vi "IMAQController.panel2.vi"(0 "object ref":refnum<vi>, 5 "error in (no error)":errorcluster) -> ()   [LabVIEW 2014]
doc: "This is the front panel VI for the PTScanner class.\n\ndescriptionHelpStart\nThe PTScanner class has been designed to be used interactively by a normal user. The main aim of this class is to provide a possibility of multi-dimensional scan for any integer or floating-point single value among the CS system.\n\nAt first, user has to add values to be scanned and to organize them in the corresponding order. Each value is represented by several parameters:\n- object\n- \"set\" method (can have many parameters)\n- method parameters (with one of them to be scanned)\n- central point\n- \"minus\" and \"plus\" values (start point is a difference between \"central\" and \"minus\" values, stop point is a sum of \"central\" and \"plus\" respectively)\n- step size\n- call mode which means how will be realized the movement from one step to the next one. The check of nominal (from current step) and actual values conformity can be done in a simple mode (here you should know the corresponding service) or in a synchronous mode (assuming that the method has a feedback of excatly the same parameters as input parameters)\n- as an option one can input service address for the synchronization directly. Do it only if you know exactly what is it!!!\n\nAfter the list of values is formed you have to form the scan sequence. You can check the scan sequence by \"View -> Scan Table\" from the window menu (have to wait some time before the representation table will be formed). Now you can run your scan in two modes: single (sequence will be runned only once) and loop (sequence will be runned continuously).\n\nDelay is a delay time (in ms) between two steps.\ndescriptionHelpStop\n\nLicense Agreement for the PTScanner class:\n\nCopyright (C)\nMikhail Goncharov\nMax-Planck-Institut fuer Kernphysik\nSaupfercheckweg 1\n69117 Heidelberg\nGermany\n\nContact: mikhail.goncharov@mpi-hd.mpg.de\n\nThis program is free software; you can redistribute it and/or modify it under the terms of the GNU General Public License as published by the Free Software Foundation; either version 2 of the license, or (at your option) any later version.\n\nThis program is distributed in the hope that it will be useful, but WITHOUT ANY WARRANTY; without even the implied warranty of MERCHANTABILITY or FITNESS FOR A PARTICULAR PURPOSE. See the GNU General License for more details (http://www.gnu.org).\n\nLast update: 2-DEC-2010\n\n\nmenuHelpStart\nFile\n==\n- \"Load\" loads a list of values to be scanned. After that you have to form a scan.\n\n- \"Save/Save As\" saves the actual list of values.\n\n- \"Hide\" just hides this GUI (but it remains alive in the background).\n\n- \"Close\" closes this window and removes this process from the system.\n\nOperate\n=====\n- \"Start\" starts scan sequence. Awailable only after the sequence is formed.\n\n- \"Pause\" pauses current run. Awailable only during the running of the sequence.\n\n- \"Stop\" stops scan sequence.\n\n- \"Reset\" resets the scanner (sets the first step as a current and nulls all counters).\n\n- \"Reset Values\" sets all variables to their central values.\n\nView\n=====\n- \"Scan Table\" forms and shows the representation of the current formed scan sequence. If there are a lot of steps and values it could take some time so be patient =)\nmenuHelpStop"
uses:
  CSlibraries-extern/DimLVEvent/DimIndicators/DimIndicators.lvlib
  CSCore/CSSystem/CSSystemLib/CSSystemLib.lvlib
  CSlibraries-extern/DimLVEvent/LVDimInterface/LVDimInterface.lvlib
  CSlibraries-extern/DimLVEvent/LVDimInterface/LVDimInterface.dim service type.ctl
  CSlibraries-extern/DimLVEvent/LVDimInterface/LVDimInterface.dic_info_service_notifier.vi
  CSCore/CSObj/CSObj.lvlib
  IMAQController.lvlib
  CSCore/BaseProcess/BaseProcess.lvlib
  CSCore/CSSystem/CoreLib/CoreLib.lvlib
  CSCore/CSSystem/CoreLib/CoreLib.short 2 byte array.vi
  CSlibraries-extern/HGF/HGF_VisionTools/HGF_VisionTools.lvlib
  CSlibraries-extern/DimLVEvent/LVDimInterface/LVDimInterface.dic_info_service_queue.vi
  CSlibraries-extern/DimLVEvent/DimIndicators/DimIndicators.numericType.ctl
  CSlibraries-extern/DimLVEvent/DimIndicators/DimIndicators.anyType.ctl
  CSlibraries-extern/DimLVEvent/DimIndicators/DimIndicators.numericArrayType.ctl
panel:
  out "Image hight":i32
  out "Image length":i32
  out "receivedCounter":i32
  out "receivedCounter 2":i32
  out "aktueller\nService":i32
  out "callBackID":i32
  out "no link":bool
  out "DIM service length / byte":i32
  out "act Time Stamp":i16[](array[numeric])
  out "2nd loop":i32
  out "accepted update 2nd loop":i32
  out "error out 3":errorcluster
  in  "error out 2":errorcluster
  out "TimeStamp Data":i16[](array[numeric])
  out "Abbruch durch Asynch":bool
  out "Abbruch?":bool
  out "accepted updates?":i32
  out "updates?":i32
  out "TimeStamp Analyzer":i16[](array[numeric])
  out "Data Ana Synch?":bool
  out "floor(x/y)":i32
  in  "Limits (L:0,H:255)":cluster{u8, u8}(slide)={0, 255} scale=0.0..255.0
  in  "Grab":bool
  in  "Snap":bool
  in  "Compression mode?":bool
  out "Busy 3":bool
  out "Busy 2":bool
  in  "IMAQDevice Mode":u16(ring) caption="IMAQDevice:" items=["cam1", "cam2"]
  in  "IMAQAnalyzer:":string
  in  "NumberOfImagesLink":T1
  out "CSNodes":string[](array[string])
  out "CSSystems":string[](array[string])
  in  "TimeStampAnalyzerLink":T2
  in  "TimeStampDeviceLink":T2
  in  "IntensityLink":T1
  in  "verticalProjectionLink":T2
  in  "horizontalProjectionLink":T2
  in  "WidthLink":T1
  in  "HeightLink":T1
  in  "ActualImageLink(Compression Mode)":T3
  in  "CompressionModeLink":T1
  in  "Abort Button":bool
  in  "Stop Button":bool
  in  "Start Button":bool
  in  "Step 2":dbl caption="Step"
  in  "Dec 2":dbl caption="-"
  in  "Inc 2":dbl caption="+"
  in  "Center 2":dbl caption="Center:"
  in  "Parameter 2":u16(ring) caption="Parameter:" items=["Voltage", "Current"]
  in  "Device 2":u16(ring) caption="Device:" items=["PowerSupply 1", "Power Supply 2"]
  in  "Step 1":dbl caption="Step"
  in  "Dec 1":dbl caption="-"
  in  "Inc 1":dbl caption="+"
  in  "Center 1":dbl caption="Center:"
  in  "Parameter 1":u16(ring) caption="Parameter:" items=["Voltage", "Current"]
  in  "Device 1":u16(ring) caption="Device:" items=["PowerSupply 1", "Power Supply 2"]
  in  "Scan?":bool
  in  "2 D?":bool
  in  "GetControl":bool
  out "Controller Listbox":i32(listbox)
  out "Scan_Image":T4(plugin-control)
  out "Actual_Image":T4(plugin-control)
  in  "stop":bool
  out "loop counter":i32
  out "Paused":bool
  in  "settings path":path caption="Settings file"
  out "Error":bool
  out "ErrorString":string
  out "error out":errorcluster
  # "IMAQ Configuration"
  # "Analysis Configuration"
  # "Controller Configuration"
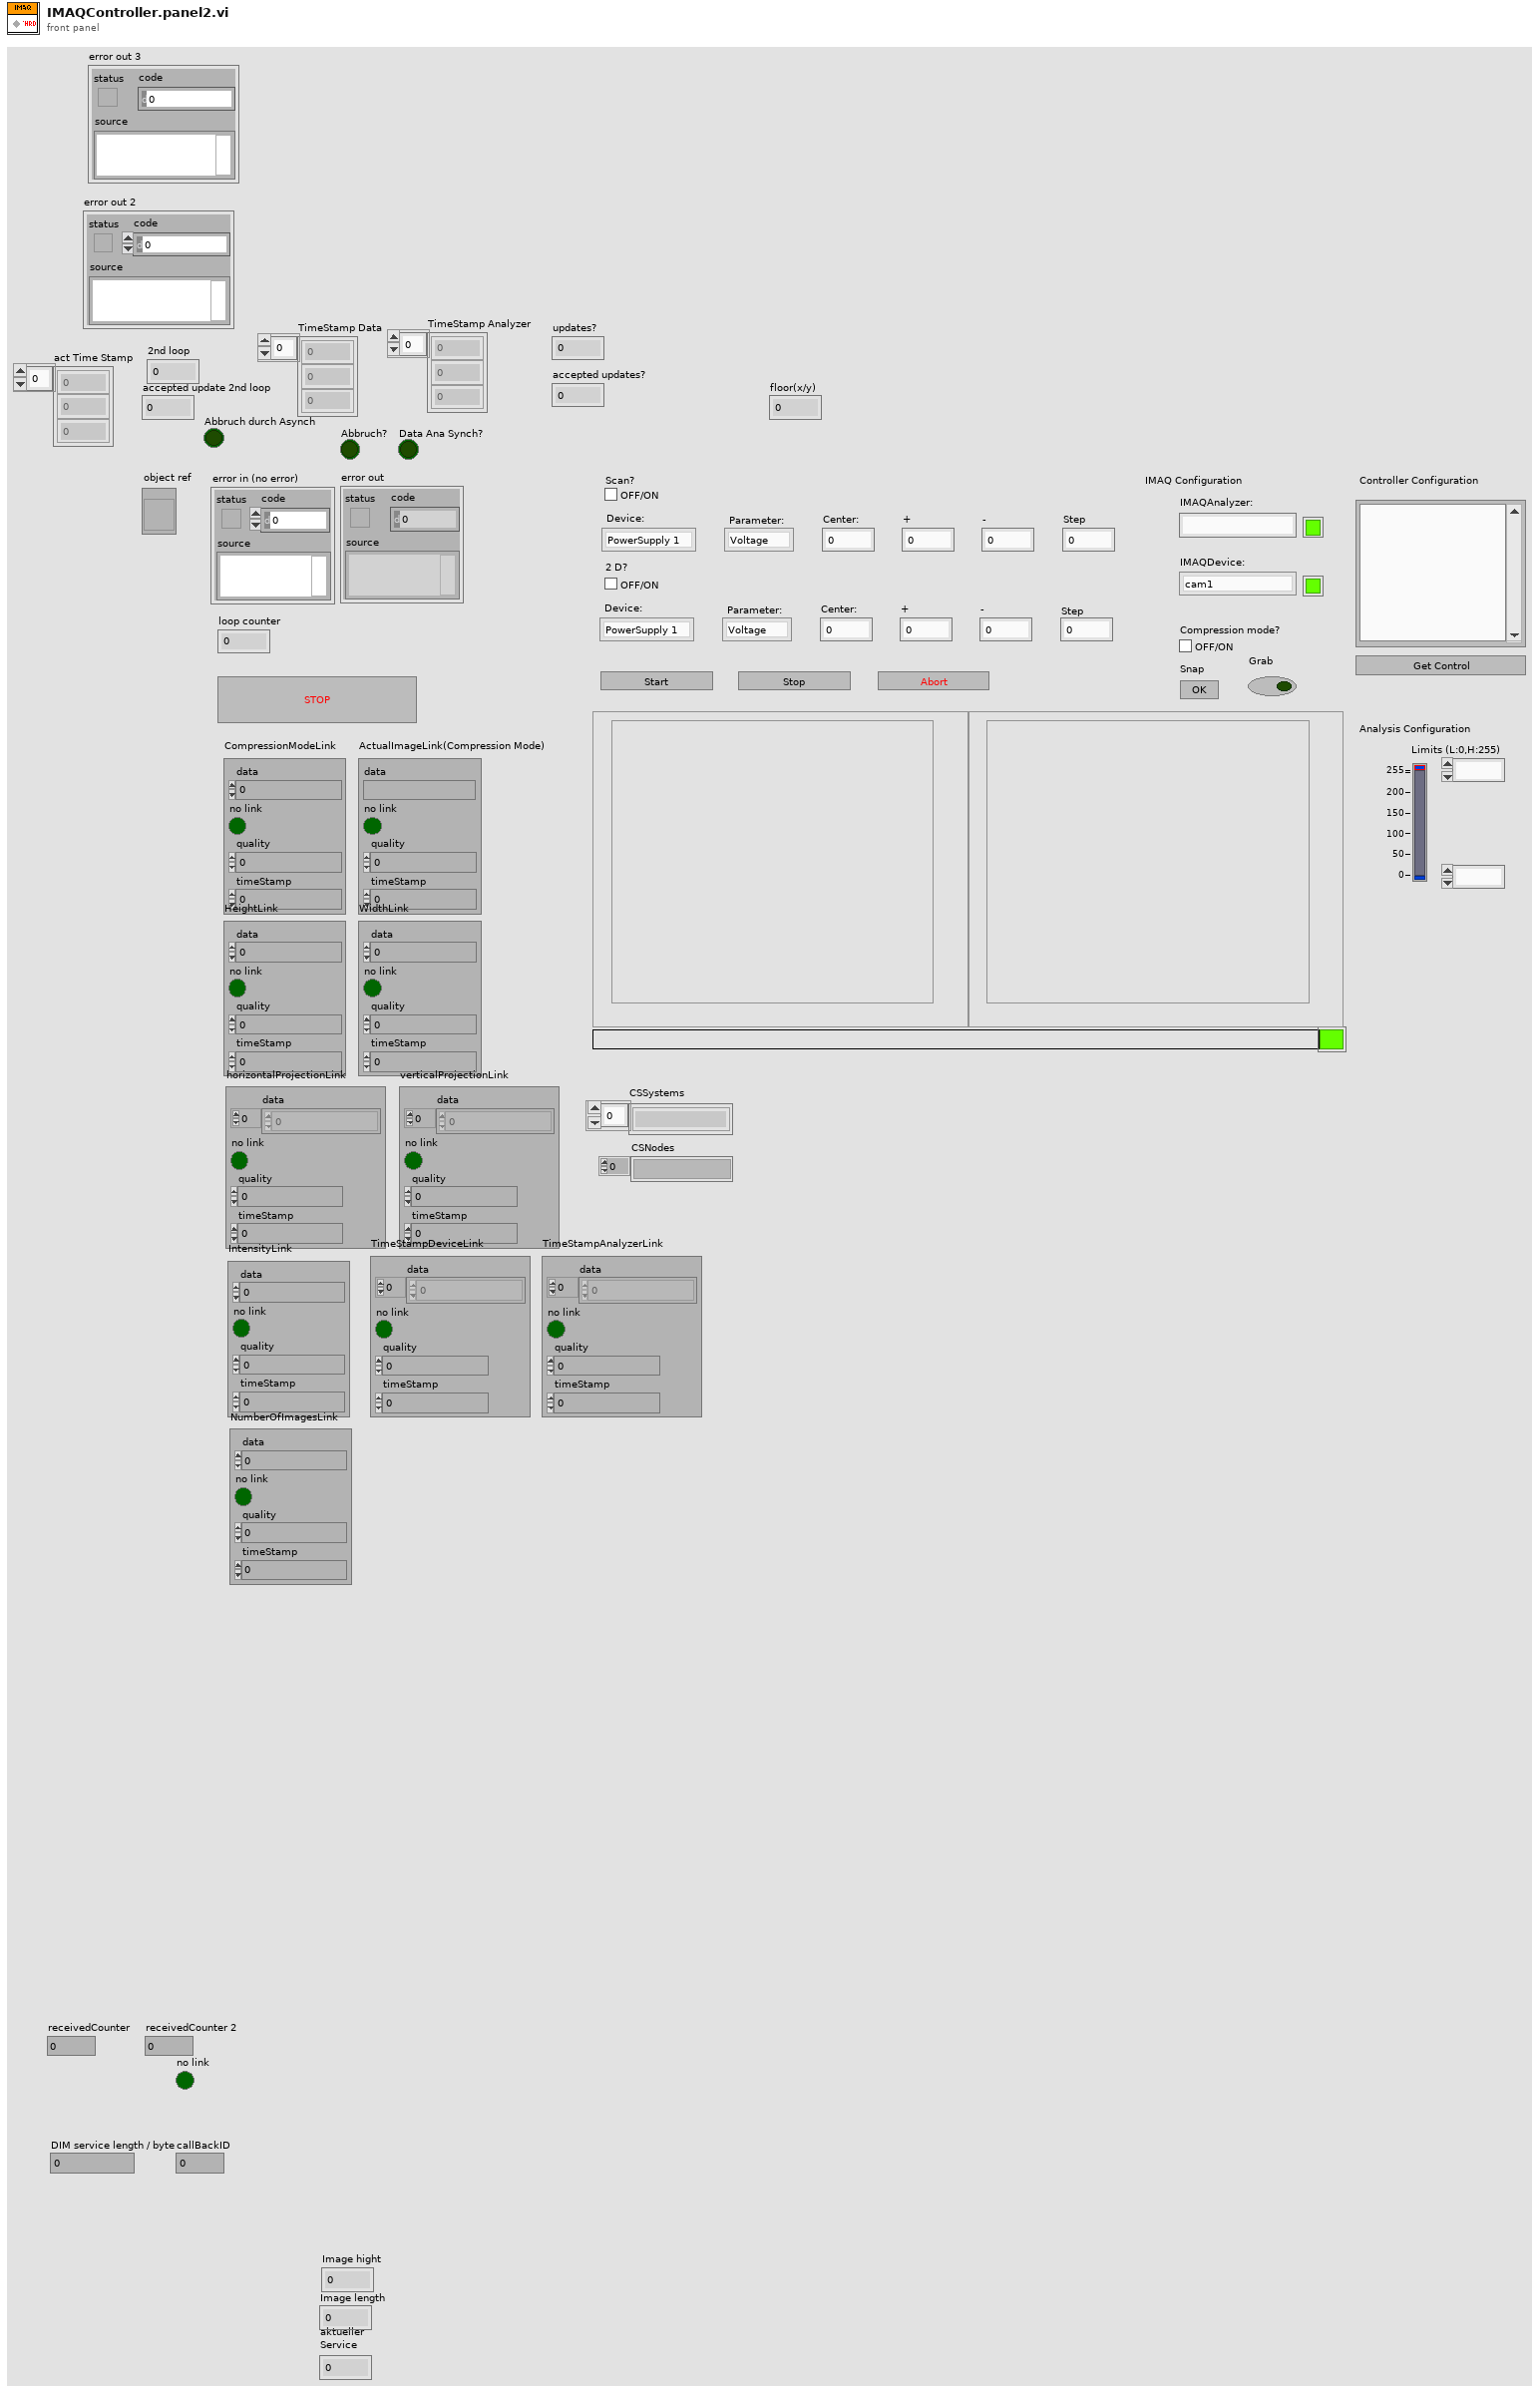
[diagram p1: front panel]
types:
  T1 = typedef "DimIndicators.lvlib/DimIndicators.numericType.ctl" = cluster{"data":dbl, "no link":bool, "quality":i32, "timeStamp":dbl}
  T2 = typedef "DimIndicators.lvlib/DimIndicators.numericArrayType.ctl" = cluster{"data":dbl[], "no link":bool, "quality":i32, "timeStamp":dbl}
  T3 = typedef "DimIndicators.lvlib/DimIndicators.anyType.ctl" = cluster{"data":string, "no link":bool, "quality":i32, "timeStamp":dbl}
  T4 = typedef "IMAQ Image.ctl" = refnum<image>
  T5 = typedef "Image Type" = u32
  T6 = typedef "IMAQController.lvlib/IMAQController.i attribute.ctl" = cluster{"ImageTakenID":i32, "actSequencer":string, "actScanner":string, "CameraTriggerID":i32, "activatedCameras":cluster{"Name":string, "Camera Type":string, "Acquisition Mode":u32, "JPEG Mode?":bool, "Acquisition Delay":dbl, "Save Images?":bool, "Center Coordinates":T7, "PixelPermm":cluster{"Horizontal":dbl, "Vertical":dbl}, "Rotation":dbl, "Mirror Mode":u32, "PixelCoordinates":cluster{"1":cluster{"Horizontal":i32, "Vertical":i32}, "2":cluster{"Horizontal":i32, "Vertical":i32}, "3":cluster{"Horizontal":i32, "Vertical":i32}, "4":cluster{"Horizontal":i32, "Vertical":i32}}, "RWCoordinates":cluster{"1":cluster{"Horizontal":dbl, "Vertical":dbl}, "2":cluster{"Horizontal":dbl, "Vertical":dbl}, "3":cluster{"Horizontal":dbl, "Vertical":dbl}, "4":cluster{"Horizontal":dbl, "Vertical":dbl}}, "HorizScaling":dbl, "VertScaling":dbl}[], "Ini C-Array":string[], "actCamera":string, "activeCamera":cluster{"Name":string, "Camera Type":string, "Aqcuisation Mode":enum32{"Internal Trigger", "Scan", "free Running", "External Trigger"}, "JPEG Mode?":bool, "Acquisition Delay":dbl, "Save Images?":bool, "Center Coordinates":T7, "PixelPermm":cluster{"Horizontal":dbl, "Vertical":dbl}, "Rotation":dbl, "Mirror Mode":u32, "PixelCoordinates":cluster{"1":cluster{"Horizontal":i32, "Vertical":i32}, "2":cluster{"Horizontal":i32, "Vertical":i32}, "3":cluster{"Horizontal":i32, "Vertical":i32}, "4":cluster{"Horizontal":i32, "Vertical":i32}}, "RWCoordinates":cluster{"1":cluster{"Horizontal":dbl, "Vertical":dbl}, "2":cluster{"Horizontal":dbl, "Vertical":dbl}, "3":cluster{"Horizontal":dbl, "Vertical":dbl}, "4":cluster{"Horizontal":dbl, "Vertical":dbl}}, "HorizScaling":dbl, "VertScaling":dbl}, "BilderMittelungen":u8, "OldPicture":dbl[][]}
  T7 = typedef "LVPoint32TypeDef.ctl" = cluster{"Horizontal":i32, "Vertical":i32}
  T8 = enum8{"Enabled", "Disabled", "Disabled and Grayed Out"}
  T9 = typedef "LVDimInterface.lvlib/LVDimInterface.dim service type.ctl" = u16
  T10 = typedef "CoreDefs.rawDataType.ctl" = i8[]
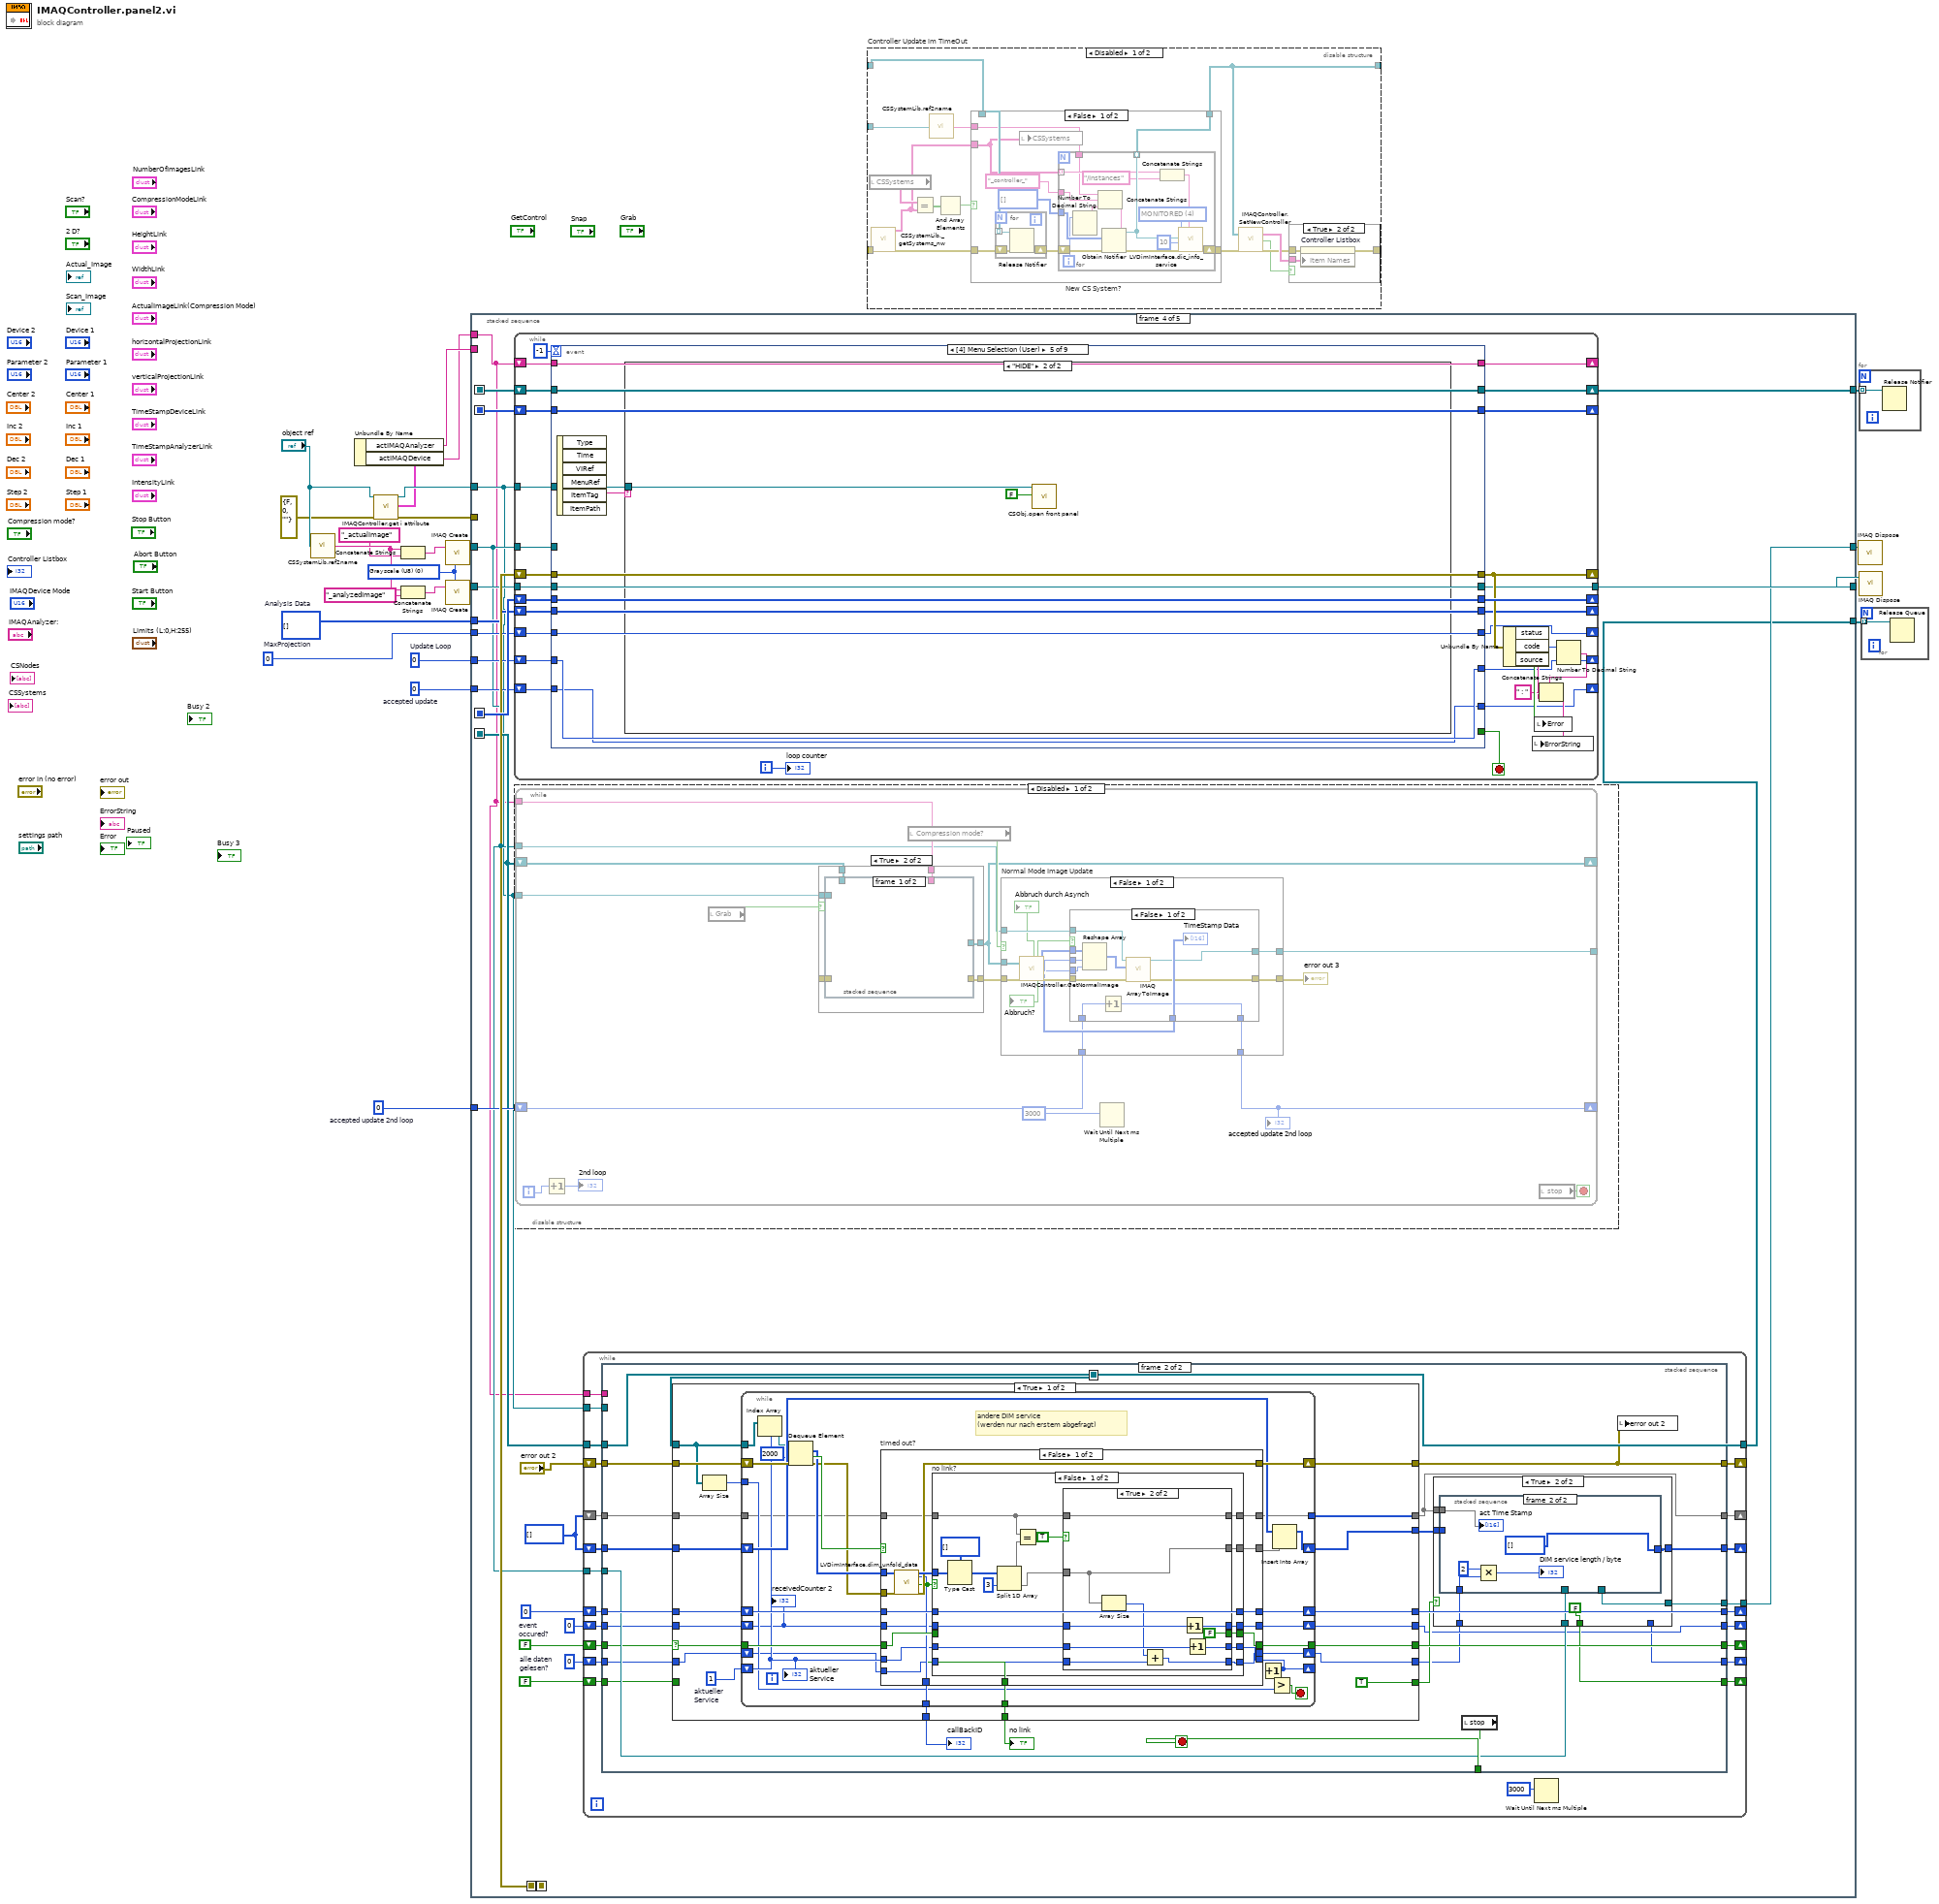
[diagram p0: block diagram]
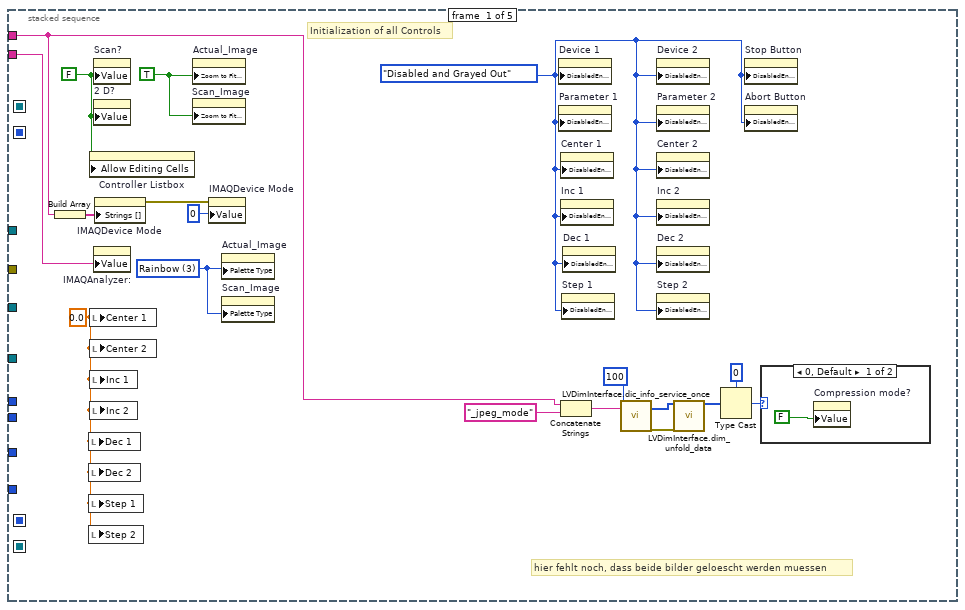
[diagram p5: hidden frame]
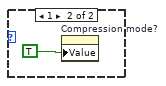
[diagram p6: hidden frame]
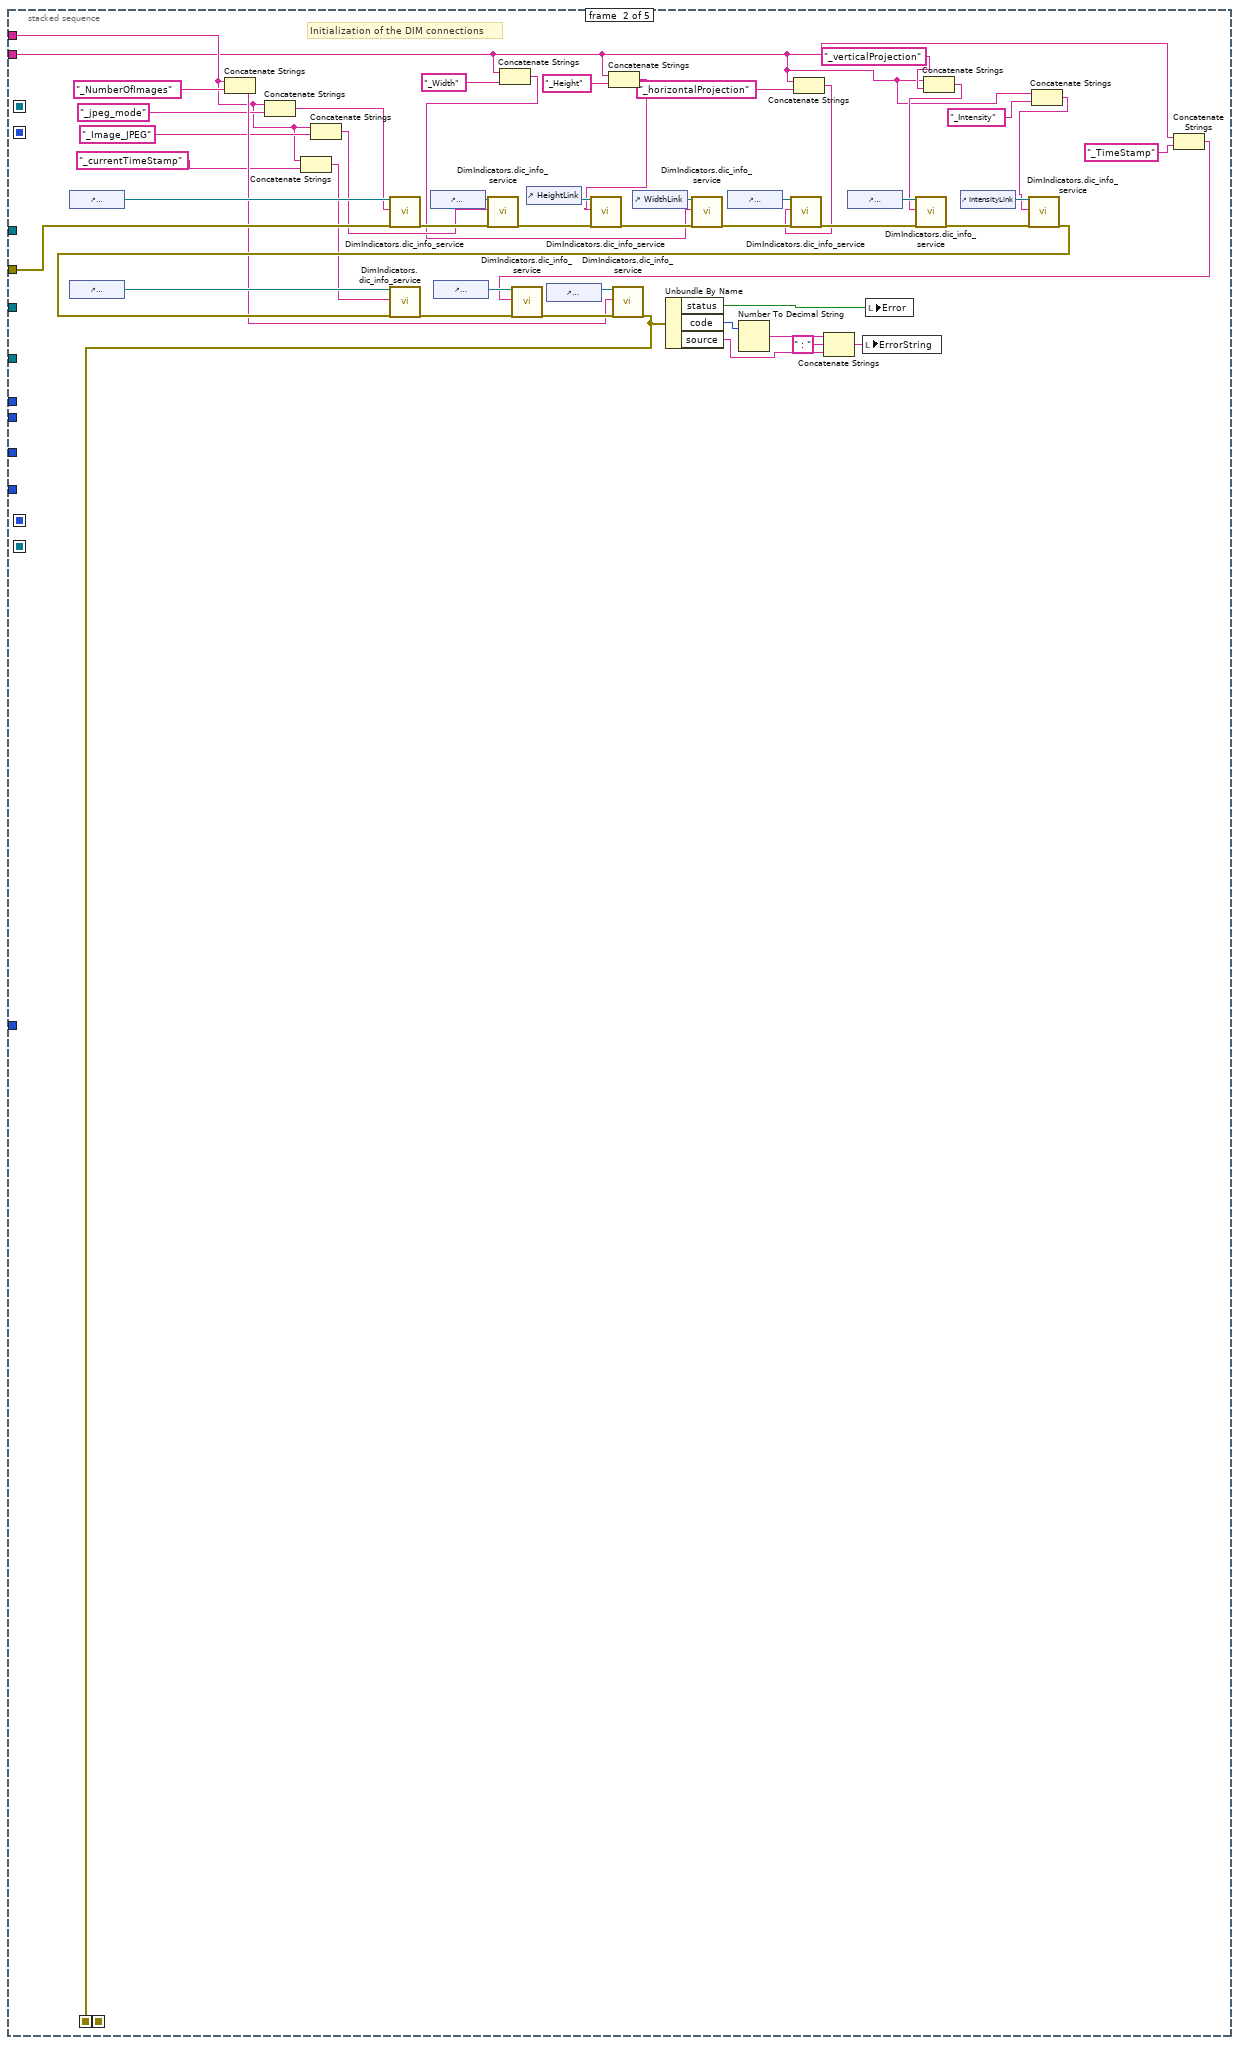
[diagram p7: hidden frame]
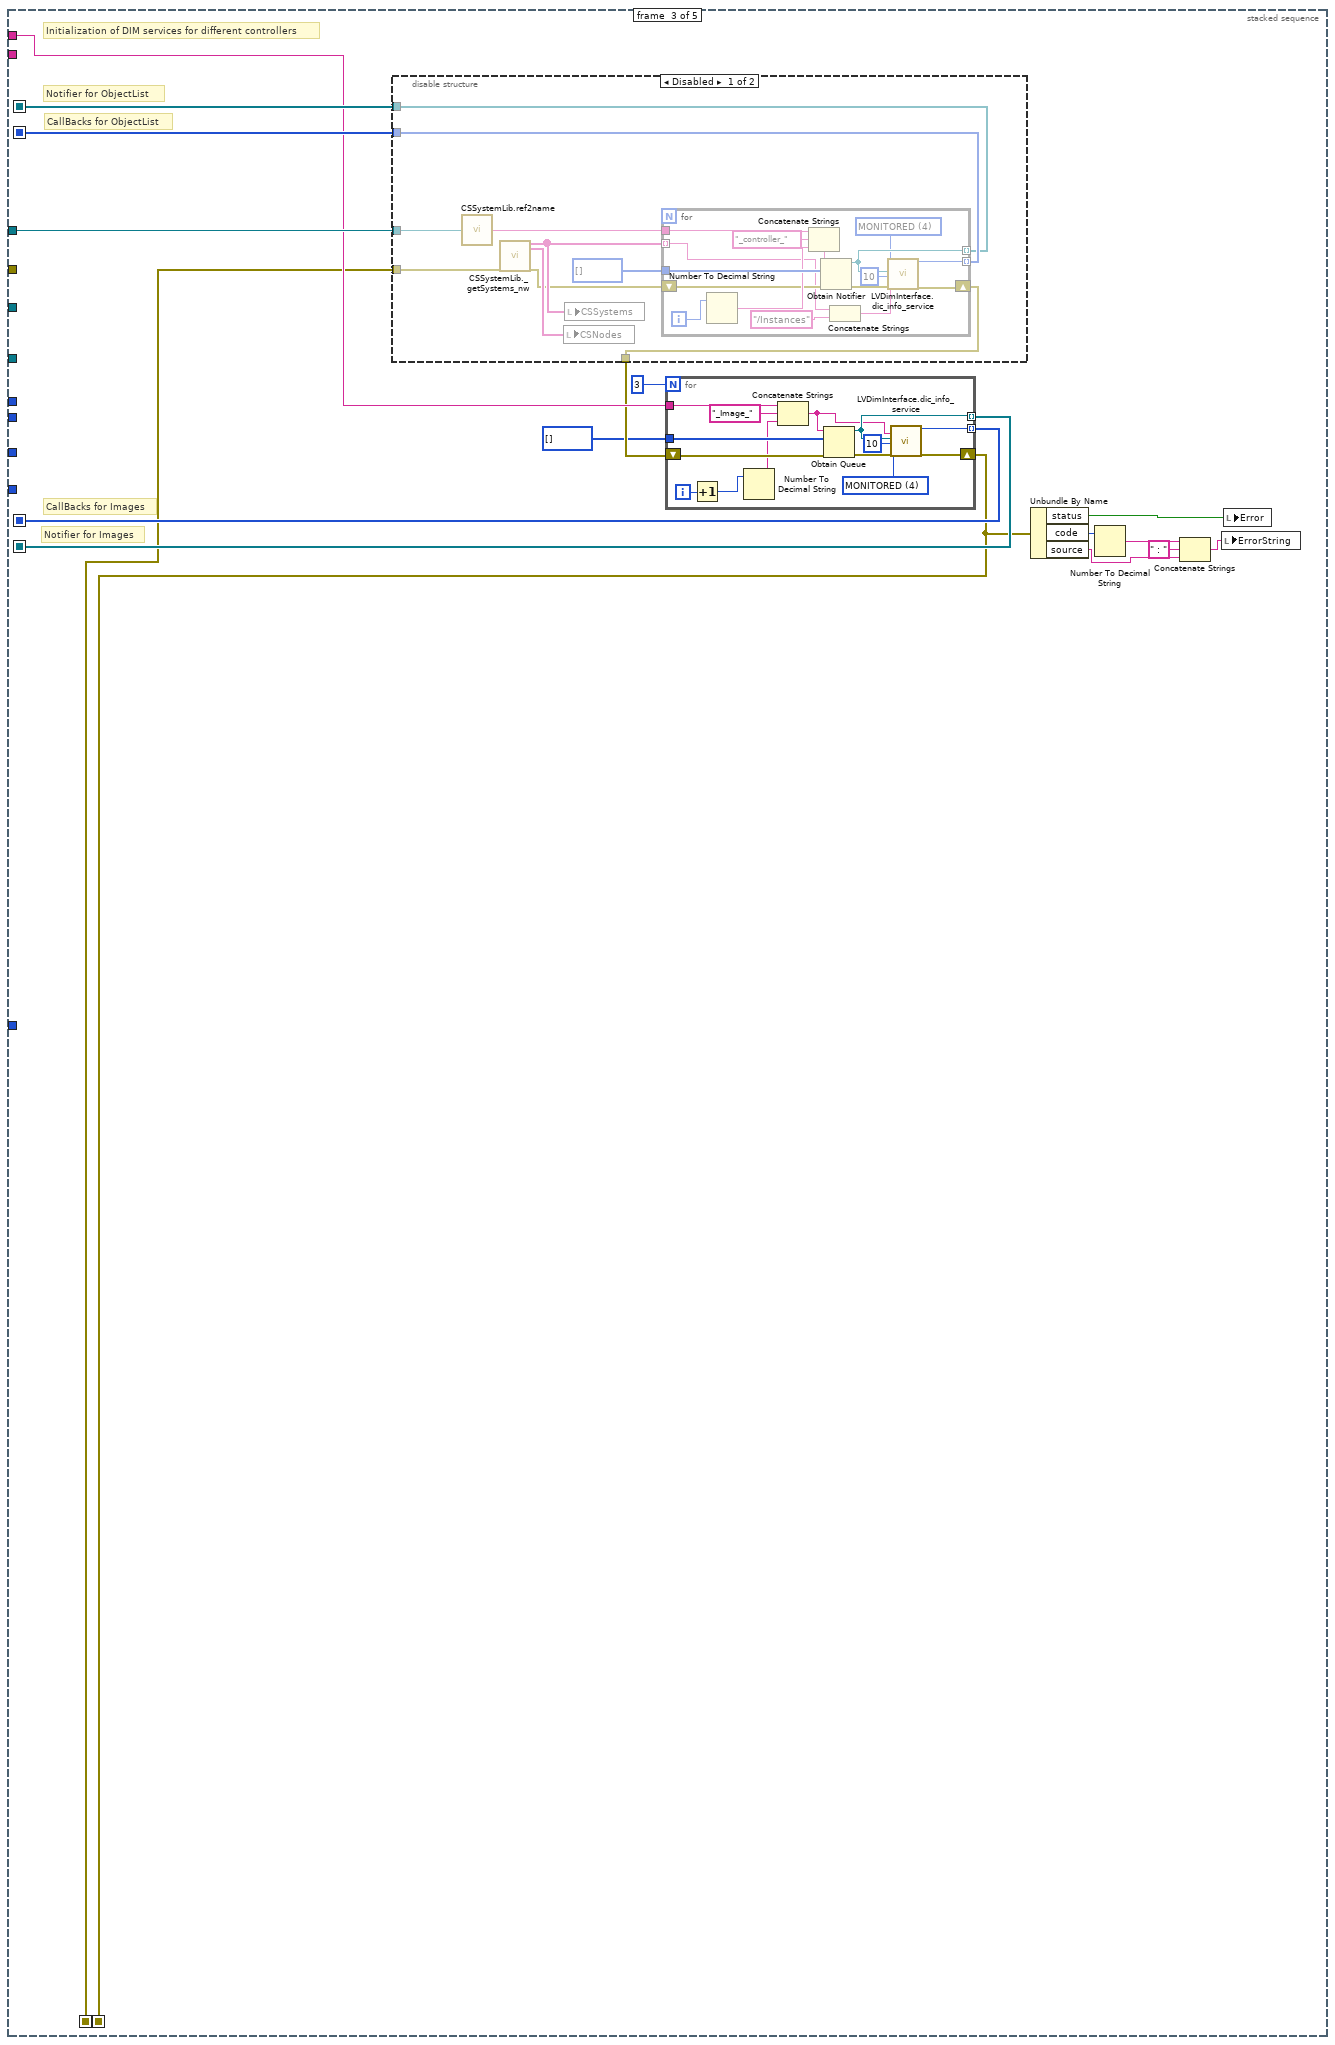
[diagram p8: hidden frame]
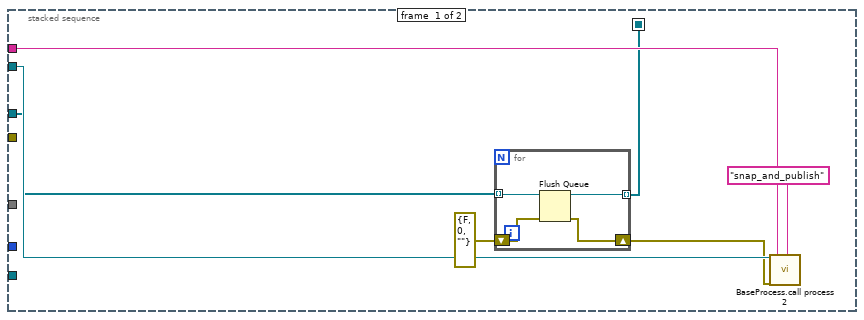
[diagram p10: hidden frame]
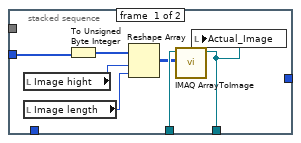
[diagram p12: hidden frame]
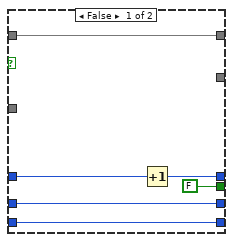
[diagram p13: hidden frame]
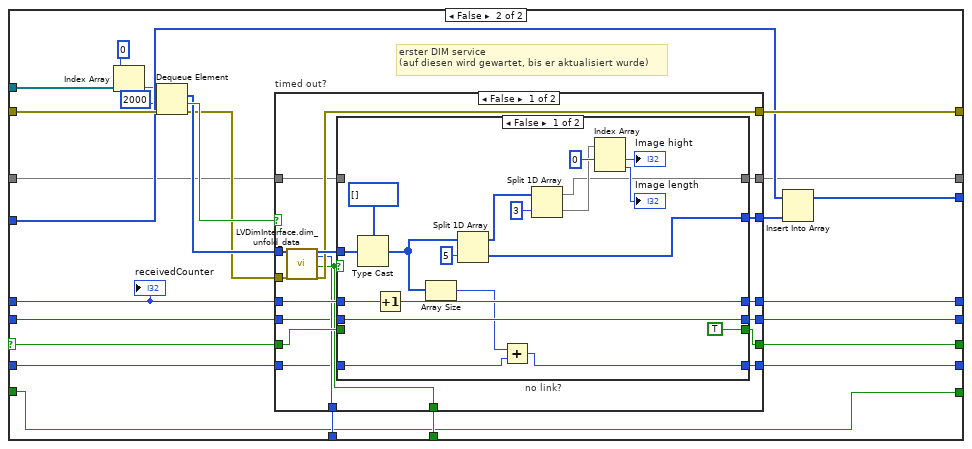
[diagram p16: hidden frame]
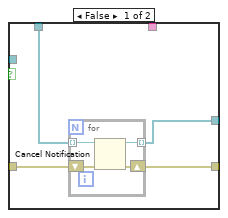
[diagram p19: hidden frame]
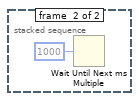
[diagram p20: hidden frame]
diagram:
  w1 = 0  # accepted update 2nd loop
  w5 = 0  # accepted update
  w4 = 0  # Update Loop
  w6 = 0  # MaxProjection
  w7 = u8[][] []  # Analysis Data
  w24 = T5 0 items=["Grayscale (U8)", "Grayscale (I16)", "Grayscale (SGL)", "Complex (CSG)", "RGB (U32)", "HSL (U32)", "RGB (U64)", "Grayscale (U16)"] ("Image Type")
  n1 = call "CSSystemLib.ref2name.vi"("obj refnum"="object ref") -> ("name"=w21:string)
  n2 = call "IMAQController.get i attribute.vi"("i ref in"="object ref", "error in (no error)"=errorcluster {"status"=FALSE, "code"=0, "source"=""}) -> ("i ref out"=w15:refnum<vi>, "i attribute"=w12:T6, "error out"=w13:errorcluster)  [unwired: 15 in]
  n3 = Unbundle By Name(w12) -> ("actIMAQAnalyzer"=w11:string, "actIMAQDevice"=w10:string)
  n4 = Concatenate Strings(w21, "_actualImage" ("string")) -> (w22:string)
  n5 = Concatenate Strings(w21, "_analyzedImage" ("string")) -> (w23:string)
  n6 = call "IMAQ Create"("Image Name"=w22, "Image Type"=w24) -> ("New Image"=w18:T4)  [unwired: 3 in, 1 out]
  n7 = call "IMAQ Create"("Image Name"=w23, "Image Type"=w24) -> ("New Image"=w9:T4)  [unwired: 3 in, 1 out]
  n8 = stacked-sequence {
    seq-local: [_ _ w110 _ _] -> [_ _ _ w174 w783]
    seq-local: [_ _ w109 _ _] -> [_ _ _ w175 _]
    seq-local: [_ _ w108 _ _] -> [_ _ _ w158 _]
    seq-local: [_ _ w107 _ _] -> [_ _ _ w176 w782]
    seq-local: [_ w51 _ _ _] -> [_ _ w104 _ _]
    seq-local: [_ _ w103 _ _] -> [_ _ _ w173 _]
    tunnel: w15 -> [_ _ w106 w153 w784]
    tunnel: w13 -> [_ w93 _ _ _]
    tunnel: w18 -> [_ _ _ w156 _]
    tunnel: [_ _ _ w155 _] -> w17
    tunnel: w10 -> [w33 w66 w105 w152 _]
    tunnel: w11 -> [w36 w53 _ _ _]
    tunnel: w9 -> [_ _ _ w172 _]
    tunnel: [_ _ _ w171 _] -> w8
    tunnel: w7 -> [_ _ _ w170 _]
    tunnel: w6 -> [_ _ _ w169 _]
    tunnel: w5 -> [_ _ _ w168 _]
    tunnel: w4 -> [_ _ _ w167 _]
    tunnel: [_ _ _ w154 _] -> w3
    tunnel: [_ _ _ w166 _] -> w2
    tunnel: w1 -> [_ _ _ w165 _]
    frame #0 {
      w26 = u32 3 items=["Grayscale", "Binary", "Gradient", "Rainbow", "Temperature", "User Defined"] ("Palette:Palette Type")
      w25 = TRUE ("Zoom to Fit Mode")
      w41 = 0.0 ("Center 1")
      w42 = T8."Disabled and Grayed Out" ("Disabled")
      w40 = FALSE ("Scan?")
      # "hier fehlt noch, dass beide bilder geloescht werden muessen"
      # "Initialization of all Controls"
      n9 = Build Array(w33) -> (w37:string[])
      n10 = local write "Dec 1"(w41) -> ()
      n11 = local write "Dec 2"(w41) -> ()
      n12 = local write "Step 1"(w41) -> ()
      n13 = local write "Step 2"(w41) -> ()
      n14 = property on="Controller Listbox" class="LstBox (strict)"("Allow Editing Cells"=w40) -> ()  [unwired: 2 in, 2 out]
      n15 = local write "Center 1"(w41) -> ()
      n16 = local write "Center 2"(w41) -> ()
      n17 = local write "Inc 1"(w41) -> ()
      n18 = local write "Inc 2"(w41) -> ()
      n19 = property on="Scan?" class="Bool (strict)"("Value"=w40) -> ()  [unwired: 2 in, 2 out]
      n20 = property on="2 D?" class="Bool (strict)"("Value"=w40) -> ()  [unwired: 2 in, 2 out]
      n21 = property on="IMAQAnalyzer:" class="Str"("Value"=w36) -> ()  [unwired: 2 in, 2 out]
      n22 = property on="IMAQDevice Mode" class="Ring (strict)"("Strings []"=w37) -> (error out=w39:errorcluster)  [unwired: 2 in, 1 out]
      n23 = property on="Actual_Image"("Zoom to Fit Mode"=w25) -> ()  [unwired: 2 in, 2 out]
      n24 = property on="Scan_Image"("Zoom to Fit Mode"=w25) -> ()  [unwired: 2 in, 2 out]
      n25 = property on="IMAQDevice Mode" class="Ring (strict)"(error in=w39, "Value"=0) -> ()  [unwired: 1 in, 2 out]
      n26 = property on="Actual_Image"("Palette Type"=w26) -> ()  [unwired: 2 in, 2 out]
      n27 = property on="Scan_Image"("Palette Type"=w26) -> ()  [unwired: 2 in, 2 out]
      n28 = property on="Device 1" class="Ring (strict)"("DisabledEnum"=w42) -> ()  [unwired: 2 in, 2 out]
      n29 = property on="Parameter 1" class="Ring (strict)"("DisabledEnum"=w42) -> ()  [unwired: 2 in, 2 out]
      n30 = property on="Center 1" class="DigNum (strict)"("DisabledEnum"=w42) -> ()  [unwired: 2 in, 2 out]
      n31 = property on="Inc 1" class="DigNum (strict)"("DisabledEnum"=w42) -> ()  [unwired: 2 in, 2 out]
      n32 = Concatenate Strings(w33, "_jpeg_mode" ("string")) -> (w34:string)
      n33 = property on="Step 1" class="DigNum (strict)"("DisabledEnum"=w42) -> ()  [unwired: 2 in, 2 out]
      n34 = property on="Dec 1" class="DigNum (strict)"("DisabledEnum"=w42) -> ()  [unwired: 2 in, 2 out]
      n35 = call "LVDimInterface.dic_info_service_once.vi"("serviceName"=w34, "timeout [ms]"=u32 100) -> ("data"=w30:i8[], "error out"=w31:errorcluster)  [unwired: 14 in, 2 out]
      n36 = property on="Device 2" class="Ring (strict)"("DisabledEnum"=w42) -> ()  [unwired: 2 in, 2 out]
      n37 = property on="Parameter 2" class="Ring (strict)"("DisabledEnum"=w42) -> ()  [unwired: 2 in, 2 out]
      n38 = property on="Center 2" class="DigNum (strict)"("DisabledEnum"=w42) -> ()  [unwired: 2 in, 2 out]
      n39 = property on="Inc 2" class="DigNum (strict)"("DisabledEnum"=w42) -> ()  [unwired: 2 in, 2 out]
      n40 = property on="Dec 2" class="DigNum (strict)"("DisabledEnum"=w42) -> ()  [unwired: 2 in, 2 out]
      n41 = property on="Step 2" class="DigNum (strict)"("DisabledEnum"=w42) -> ()  [unwired: 2 in, 2 out]
      n42 = call "LVDimInterface.dim_unfold_data.vi"("rawData"=w30, "error in (no error)"=w31) -> ("data"=w29:i8[])  [unwired: 14 in, 3 out]
      n43 = Type Cast(type=i16 0, x=w29) -> (*(type *) &x=w27:i16)
      n44 = property on="Stop Button" class="Bool"("DisabledEnum"=w42) -> ()  [unwired: 2 in, 2 out]
      n45 = property on="Abort Button" class="Bool"("DisabledEnum"=w42) -> ()  [unwired: 2 in, 2 out]
      n46 = case shown="0, Default" w27 {
        frame 0, Default {
          n47 = property on="Compression mode?" class="Bool (strict)"("Value"=FALSE) -> ()  [unwired: 2 in, 2 out]
        }
        frame 1 {
          n48 = property on="Compression mode?" class="Bool (strict)"("Value"=TRUE) -> ()  [unwired: 2 in, 2 out]
        }
      }
    }
    frame #1 {
      # "Initialization of the DIM connections"
      n49 = control-ref of="CompressionModeLink"() -> (w92:refnum<vi>)
      n50 = control-ref of="TimeStampDeviceLink"() -> (w82:refnum<vi>)
      n51 = Concatenate Strings(w66, "_NumberOfImages" ("string")) -> (w73:string)
      n52 = Concatenate Strings(w66, "_jpeg_mode" ("string")) -> (w70:string)
      n53 = Concatenate Strings(w66, "_currentTimeStamp" ("string")) -> (w65:string)
      n54 = Concatenate Strings(w66, "_Image_JPEG" ("string")) -> (w68:string)
      n55 = call "DimIndicators.dic_info_service.vi"("controlRef"=w92, "serviceName"=w70, "error in (no error)"=w93) -> ("error out"=w91:errorcluster)  [unwired: 15 in, 1 out]
      n56 = control-ref of="ActualImageLink(Compression Mode)"() -> (w90:refnum<vi>)
      n57 = control-ref of="TimeStampAnalyzerLink"() -> (w79:refnum<vi>)
      n58 = call "DimIndicators.dic_info_service.vi"("controlRef"=w90, "serviceName"=w68, "error in (no error)"=w91) -> ("error out"=w89:errorcluster)  [unwired: 15 in, 1 out]
      n59 = Concatenate Strings(w53, "_Width" ("string")) -> (w63:string)
      n60 = control-ref of="HeightLink"() -> (w88:refnum<vi>)
      n61 = control-ref of="NumberOfImagesLink"() -> (w74:refnum<vi>)
      n62 = Concatenate Strings(w53, "_Height" ("string")) -> (w61:string)
      n63 = call "DimIndicators.dic_info_service.vi"("controlRef"=w88, "serviceName"=w61, "error in (no error)"=w89) -> ("error out"=w87:errorcluster)  [unwired: 15 in, 1 out]
      n64 = control-ref of="WidthLink"() -> (w86:refnum<vi>)
      n65 = call "DimIndicators.dic_info_service.vi"("controlRef"=w86, "serviceName"=w63, "error in (no error)"=w87) -> ("error out"=w85:errorcluster)  [unwired: 15 in, 1 out]
      n66 = control-ref of="horizontalProjectionLink"() -> (w78:refnum<vi>)
      n67 = Concatenate Strings(w53, "_horizontalProjection" ("string")) -> (w59:string)
      n68 = call "DimIndicators.dic_info_service.vi"("controlRef"=w78, "serviceName"=w59, "error in (no error)"=w85) -> ("error out"=w77:errorcluster)  [unwired: 15 in, 1 out]
      n69 = control-ref of="verticalProjectionLink"() -> (w76:refnum<vi>)
      n70 = Concatenate Strings(w53, "_verticalProjection" ("string")) -> (w57:string)
      n71 = call "DimIndicators.dic_info_service.vi"("controlRef"=w76, "serviceName"=w57, "error in (no error)"=w77) -> ("error out"=w84:errorcluster)  [unwired: 15 in, 1 out]
      n72 = control-ref of="IntensityLink"() -> (w83:refnum<vi>)
      n73 = Concatenate Strings(w53, "_Intensity" ("string")) -> (w55:string)
      n74 = call "DimIndicators.dic_info_service.vi"("controlRef"=w83, "serviceName"=w55, "error in (no error)"=w84) -> ("error out"=w81:errorcluster)  [unwired: 15 in, 1 out]
      n75 = call "DimIndicators.dic_info_service.vi"("controlRef"=w82, "serviceName"=w65, "error in (no error)"=w81) -> ("error out"=w80:errorcluster)  [unwired: 15 in, 1 out]
      n76 = Concatenate Strings(w53, "_TimeStamp" ("string")) -> (w52:string)
      n77 = call "DimIndicators.dic_info_service.vi"("controlRef"=w79, "serviceName"=w52, "error in (no error)"=w80) -> ("error out"=w75:errorcluster)  [unwired: 15 in, 1 out]
      n78 = call "DimIndicators.dic_info_service.vi"("controlRef"=w74, "serviceName"=w73, "error in (no error)"=w75) -> ("error out"=w51:errorcluster)  [unwired: 15 in, 1 out]
      n79 = Unbundle By Name(w51) -> ("status"=w50:bool, "code"=w49:i32, "source"=w47:string)
      n80 = Number To Decimal String(number=w49) -> (decimal integer string=w48:string)  [unwired: 1 in]
      n81 = Concatenate Strings(w48, " : " ("string"), w47) -> (w45:string)
      n82 = local write "ErrorString"(w45) -> ()
      n83 = local write "Error"(w50) -> ()
    }
    frame #2 {
      # "CallBacks for Images"
      # "Notifier for Images"
      # "CallBacks for ObjectList"
      # "Notifier for ObjectList"
      # "Initialization of DIM services for different controllers"
      n84 = disable-structure shown="Disabled" {
        disable-tunnel: [w120 _] -> w110
        disable-tunnel: [w119 _] -> w109
        disable-tunnel: w106 -> [w118 _]
        disable-tunnel: w104 -> [w117 w137]
        disable-tunnel: [w113 w137] -> w101
        frame Disabled {
          n85 = call "CSSystemLib.ref2name.vi"("obj refnum"=w118) -> ("name"=w111:string)
          n86 = call "CSSystemLib._getSystems_nw.vi"("error in (no error)"=w117) -> ("CSSystems"=w116:string[], "CSNodes"=w115:string[], "error out"=w114:errorcluster)  [unwired: 16 in]
          n87 = local write "CSNodes"(w115) -> ()
          n88 = local write "CSSystems"(w116) -> ()
          n89 = for {
            tunnel: w116 -> [w123] mode=indexing
            tunnel: i8[] [] -> [w136]
            shift-right: [w129] -> w113
            shift-left: w114 -> [w131]
            tunnel: [w128] -> w119 mode=indexing
            tunnel: [w125] -> w120 mode=indexing
            tunnel: w111 -> [w121]
            i -> [w135]
            w126 = T9 4 items=["ONCE_ONLY"=1, "TIMED"=2, "MONITORED"=4] ("serviceType")
            n90 = Number To Decimal String(number=w135) -> (decimal integer string=w134:string)  [unwired: 1 in]
            n91 = Concatenate Strings(w121, "_controller_" ("string"), w134) -> (w132:string)
            n92 = Obtain Notifier(name (unnamed)=w132, notification data type=w136, error in (no error)=w131) -> (notifier out=w128:refnum<notifier>, error out=w130:errorcluster)  [unwired: 1 in, 1 out]
            n93 = Concatenate Strings(w123, "/Instances" ("string")) -> (w124:string)
            n94 = call-poly "LVDimInterface.dic_info_service.vi"("serviceName"=w124, "notifierRef"=w128, "timeout [s]"=10, "serviceType"=w126, "error in (no error)"=w130) -> ("callBackID"=w125:i32, "error out"=w129:errorcluster)  [unwired: 13 in]
          }
        }
        frame Enabled {
        }
      }
      n95 = for {
        N: 3 -> [_]
        shift-right: [w149] -> w103
        shift-left: w101 -> [w151]
        tunnel: i8[] [] -> [w148]
        tunnel: [w147] -> w108 mode=indexing
        tunnel: [w146] -> w107 mode=indexing
        tunnel: w105 -> [w143]
        i -> [w145]
        w140 = T9 4 items=["ONCE_ONLY"=1, "TIMED"=2, "MONITORED"=4] ("serviceType")
        n96 = Increment(x=w145) -> (x+1=w144:i32)
        n97 = Number To Decimal String(number=w144) -> (decimal integer string=w142:string)  [unwired: 1 in]
        n98 = Concatenate Strings(w143, "_Image_" ("string"), w142) -> (w138:string)
        n99 = Obtain Queue(name (unnamed)=w138, element data type=w148, error in (no error)=w151) -> (queue out=w147:refnum<queue>, error out=w150:errorcluster)  [unwired: 2 in, 1 out]
        n100 = call-poly "LVDimInterface.dic_info_service.vi"("serviceName"=w138, "queueRef"=w147, "timeout [s]"=10, "serviceType"=w140, "error in (no error)"=w150) -> ("callBackID"=w146:i32, "error out"=w149:errorcluster)  [unwired: 13 in]
      }
      n101 = Unbundle By Name(w103) -> ("status"=w100:bool, "code"=w97:i32, "source"=w96:string)
      n102 = Number To Decimal String(number=w97) -> (decimal integer string=w99:string)  [unwired: 1 in]
      n103 = Concatenate Strings(w99, " : " ("string"), w96) -> (w95:string)
      n104 = local write "ErrorString"(w95) -> ()
      n105 = local write "Error"(w100) -> ()
    }
    frame #3 {
      w159 = i16[] []
      w162 = FALSE  # alle daten gelesen?
      w163 = FALSE  # event  occured?
      n106 = while {
        shift-right: [w534] -> _
        shift-left: w173 -> [w544]
        tunnel: w156 -> [w543]
        shift-right: [w540] -> _
        shift-left: w176 -> [w542]
        shift-right: [w537] -> w166
        shift-left: w175 -> [w539]
        shift-right: [w536] -> _
        shift-left: w174 -> [w538]
        tunnel: w153 -> [w535]
        shift-right: [w526] -> _
        shift-left: w152 -> [w527]
        tunnel: w172 -> [w525]
        tunnel: [w524] -> w171
        shift-right: [w522] -> _
        shift-left: w170 -> [w523]
        shift-right: [w520] -> _
        shift-left: w169 -> [w521]
        shift-right: [w517] -> _
        shift-left: w167 -> [w519]
        shift-right: [w516] -> _
        shift-left: w168 -> [w518]
        i -> [w545]
        stop <- w546 stop-if-true
        n107 = event shown="[4] Menu Selection (User)" {
          selector: _ -> [_ _ _ _ _ _ _ _ _]
          dyn-events: _ -> [_ _ _ _ _ _ _ _ _]
          timeout: -1 -> [_ _ _ _ _ _ _ _ _]
          tunnel: [_ _ _ _ _ _ _ _ "stop"] -> w546
          tunnel: w544 -> [w547 w566 w642 w662 w684 w704 w712 w745 w758]
          tunnel: [w547 w577 w644 w660 w684 w703 w711 w744 w758] -> w534
          tunnel: w543 -> [_ _ _ w661 _ _ _ _ _]
          tunnel: w542 -> [w555 w578 w647 w659 w683 w699 w713 w747 w759]
          tunnel: [w555 w578 w647 w659 w683 w699 w713 w747 w759] -> w540
          tunnel: w539 -> [_ w581 w649 w658 w686 w697 w715 w749 w757]
          tunnel: w538 -> [w554 w579 w648 w657 w685 w698 w714 w748 w756]
          tunnel: [_ w581 w649 w658 w686 w697 w715 w749 w757] -> w537
          tunnel: [w554 w579 w648 w657 w685 w698 w714 w748 w756] -> w536
          tunnel: w535 -> [_ _ _ _ w681 w705 _ w743 _]
          tunnel: w527 -> [w553 w580 w650 w656 w680 w696 w716 w742 w755]
          tunnel: [w553 w580 w650 w656 w680 w696 w716 w742 w755] -> w526
          tunnel: w525 -> [w552 w576 w640 w655 w679 w693 w710 w741 w754]
          tunnel: [w552 w575 w640 w655 w679 w693 w710 w741 w754] -> w524
          tunnel: w523 -> [w551 w573 w639 w654 w678 w692 w709 w740 w753]
          tunnel: [w551 w571 w639 w654 w678 w692 w709 w740 w753] -> w522
          tunnel: w521 -> [w550 w574 w638 w653 w677 w691 w708 w739 w752]
          tunnel: [w550 w572 w638 w653 w677 w691 w708 w739 w752] -> w520
          tunnel: w519 -> [w549 w561 w637 w652 w676 w690 w707 w738 w751]
          tunnel: w518 -> [w548 w558 w636 w651 w675 w689 w706 w737 w750]
          tunnel: [w549 w560 w637 w652 w676 w690 w707 w738 w751] -> w517
          tunnel: [w548 w557 w636 w651 w675 w689 w706 w737 w750] -> w516
          event Timeout {
            n108 = event-data() -> ()  [unwired: 1 in, 2 out]
          }
          event Value Change {
            n109 = event-data() -> ()  [unwired: 1 in, 5 out]
            n110 = local read "TimeStamp Data"() -> (w556:i16[])
            n111 = property on="horizontalProjectionLink" class="Clust (strict)"(error in=w566) -> (error out=w568:errorcluster, "Value"=w567:T2)  [unwired: 1 in, 1 out]
            n112 = Unbundle By Name(w567) -> ("data"=w564:dbl[])
            n113 = Split 1D Array(array=w564, index=3) -> (first subarray=w562:dbl[], second subarray=w563:dbl[])
            n114 = To Word Integer(number=w562) -> (16bit integer=w569:i16[])
            "TimeStamp Analyzer" <- w569
            n115 = Equal?(x=w569, y=w556) -> (x = y?=w570:bool[])
            n116 = And Array Elements(Boolean array=w570) -> (logical AND=w559:bool)
            "Data Ana Synch?" <- w559
            n117 = case shown="True" w559 {
              tunnel: [w586 w615] -> w577
              tunnel: w576 -> [w585 w614]
              tunnel: [w585 w613] -> w575
              tunnel: w574 -> [w588 w612]
              tunnel: w573 -> [w587 w611]
              tunnel: [w588 w610] -> w572
              tunnel: [w587 w609] -> w571
              tunnel: w568 -> [w586 w607]
              tunnel: w563 -> [_ w589]
              frame False {
              }
              frame True {
                w593 = 420 ("x")
                # "number deduced from tests\ndon't know why it is not 500..."
                n118 = Array Max & Min(array=w589) -> (max value=w602:dbl)  [unwired: 3 out]
                n119 = To Long Integer(number=w602) -> (32bit integer=w601:i32)
                n120 = Greater?(x=w601, y=w612) -> (0:w603:bool)
                n121 = case "neuen Maximalwert bestimmen" shown="True" w603 {
                  tunnel: w612 -> [w629 w632]
                  tunnel: w601 -> [_ w634]
                  tunnel: [w629 w634] -> w610
                  tunnel: w611 -> [w628 w635]
                  tunnel: [w628 w630] -> w600
                  frame False {
                  }
                  frame True {
                    n122 = Divide(x=w635, y=w634) -> (x/y=w633:dbl[][])
                    n123 = Multiply(x=w633, y=w632) -> (x*y=w631:dbl[][])
                    n124 = To Long Integer(number=w631) -> (32bit integer=w630:i32[][])
                  }
                }
                n125 = Divide(x=w589, y=w610) -> (x/y=w604:dbl[])
                n126 = Multiply(x=256, y=w604) -> (x*y=w606:dbl[])
                n127 = Insert Into Array(array=w600, new element=w606) -> (w597:i32[][])  [unwired: 2 in]
                n128 = Array Size(array=w597) -> (size(s)=w599:i32[])
                n129 = Index Array(array=w599, index=0) -> (element=w594:i32)
                n130 = Subtract(x=w593, y=w594) -> (x-y=w595:i32)
                n131 = Less Than 0?(x=w595) -> (x < 0?=w596:bool)
                n132 = case "wenn voll, alte Werte loeschen" shown="True" w596 {
                  tunnel: w597 -> [w622 w627]
                  tunnel: [w622 w626] -> w609
                  tunnel: w595 -> [_ w624]
                  frame False {
                  }
                  frame True {
                    n133 = Absolute Value(x=w624) -> (abs(x)=w623:i32)
                    n134 = Delete From Array(array=w627, length=w623, index (row)=0) -> (array with subset deleted=w626:i32[][])  [unwired: 1 in, 1 out]
                  }
                }
                n135 = Quotient & Remainder(x=w593, y=w594) -> (floor(x/y)=w592:i32)  [unwired: 1 out]
                "floor(x/y)" <- w592
                n136 = for {
                  tunnel: w609 -> [w619] mode=indexing
                  tunnel: w592 -> [w620]
                  shift-right: [w618] -> w590
                  shift-left: i32[][] [] ("Analysis Data") -> [w616]
                  n137 = for {
                    N: w620 -> [_]
                    tunnel: w619 -> [w621]
                    tunnel: [w621] -> w617 mode=indexing
                  }
                  n138 = Insert Into Array(array=w616, new element=w617) -> (w618:i32[][])  [unwired: 2 in]
                }
                n139 = call "IMAQ ArrayToImage"("error in (no error)"=w607, "Image Pixels (U8)"=w590, "Image"=w614) -> ("error out"=w608:errorcluster, "Image Out"=w613:T4)  [unwired: 7 in]
                n140 = property on="Scan_Image"(error in=w608, "Value"=w613) -> (error out=w615:errorcluster)  [unwired: 1 in, 1 out]
              }
            }
            n141 = Increment(x=w561) -> (x+1=w560:i32)
            "updates?" <- w560
            n142 = case shown="True" w559 {
              tunnel: w558 -> [w582 w584]
              tunnel: [w582 w583] -> w557
              frame False {
              }
              frame True {
                n143 = Increment(x=w584) -> (x+1=w583:i32)
              }
            }
            "accepted updates?" <- w557
          }
          event "Limits (L:0,H:255)": Value Change {
            w641 = u32 5 items=["Grayscale", "Binary", "Gradient", "Rainbow", "Temperature", "User Defined"] ("Palette:Palette Type")
            n144 = event-data() -> ("NewVal"=w646:cluster{u8, u8})  [unwired: 1 in, 4 out]
            n145 = call "ColorMap_Rainbow_LH.vi"("Limits (L:0,H:255)"=w646) -> ("Rainbow_LH"=w645:cluster{"Red":u8, "Green":u8, "Blue":u8}[])
            n146 = property on="Actual_Image"(error in=w642, "Palette Type"=w641) -> (error out=w643:errorcluster)  [unwired: 1 in, 1 out]
            n147 = property on="Actual_Image"(error in=w643, "User Palette"=w645) -> (error out=w644:errorcluster)  [unwired: 1 in, 1 out]
          }
          event Value Change {
            n148 = event-data() -> ("CtlRef"=w663:refnum<vi>, "NewVal"=w664:T3)  [unwired: 1 in, 3 out]
            n149 = local read "Compression mode?"() -> (w665:bool)
            n150 = case shown="True" w665 {
              tunnel: w664 -> [_ w674]
              tunnel: w663 -> [_ _]
              tunnel: w662 -> [w666 w672]
              tunnel: [w667 w668] -> _
              tunnel: w661 -> [w667 w671]
              tunnel: [w666 w669] -> w660
              frame False {
              }
              frame True {
                n151 = Unbundle By Name(w674) -> ("data"=w673:string)
                n152 = Unflatten From String(type=w671, binary string=w673, error in (no error)=w672) -> (value=w668:T4, error out=w670:errorcluster)  [unwired: 2 in, 1 out]
                n153 = property on="Actual_Image"(error in=w670, "Value"=w668) -> (error out=w669:errorcluster)  [unwired: 1 in, 1 out]
              }
            }
          }
          event Menu Selection (User) {
            n154 = event-data() -> ("ItemTag"=w682:string)  [unwired: 1 in, 5 out]
            n155 = case shown="\"HIDE\"" w682 {
              tunnel: w681 -> [_ w687]
              frame "False", Default {
              }
              frame "HIDE" {
                n156 = call "CSObj.open front panel.vi"("i ref in"=w687, "frontPanelOpen"=FALSE ("front panel open")) -> ()  [unwired: 16 in, 2 out]
              }
            }
          }
          event "Compression mode?": Value Change {
            n157 = event-data() -> ("NewVal"=w695:bool)  [unwired: 1 in, 4 out]
            n158 = Boolean To (0,1)(Boolean=w695) -> (0, 1=w694:i16)
            n159 = call-poly "CoreLib.data 2 byte array.vi"("i16"=w694) -> ("byteArray out"=w702:T10)  [unwired: 18 in]
            n160 = call "BaseProcess.call process 2.vi"("i ref in"=w705, "Object"=w696, "Selector"="SetJpgMode", "Data Descriptor"="S:1", "Data"=w702, "error in (no error)"=w704) -> ("error out"=w703:errorcluster)  [unwired: 12 in, 1 out]
          }
          event "IMAQDevice Mode": Mouse Down {
            n161 = event-data() -> ()  [unwired: 1 in, 7 out]
            n162 = disable-structure shown="Disabled" {
              disable-tunnel: w712 -> [w720 w736]
              disable-tunnel: [w717 w736] -> w711
              frame Disabled {
                n163 = call "CSSystemLib._getInstances_nw.vi"("error in (no error)"=w720) -> ("i list"=w722:string[], "error out"=w718:errorcluster)  [unwired: 17 in]
                n164 = for {
                  tunnel: w722 -> [w728] mode=indexing
                  shift-right: [w729] -> w719
                  shift-left: string[] [] -> [w730]
                  n165 = call "CSSystemLib.name2class_nw.vi"("name"=w728, "timeout [ms] (10000)"=u32 500) -> ("classID"=w724:string)  [unwired: 15 in, 2 out]
                  n166 = String Subset(string=w724, length (rest)=10 ("length (rest)")) -> (substring=w725:string)  [unwired: 1 in]
                  n167 = Equal?(x=w725, y="IMAQDevice") -> (x = y?=w726:bool)
                  n168 = case shown="True" w726 {
                    tunnel: w730 -> [w732 w735]
                    tunnel: [w732 w733] -> w729
                    tunnel: w728 -> [_ w734]
                    frame False {
                    }
                    frame True {
                      n169 = Insert Into Array(array=w735, new element=w734) -> (w733:string[])  [unwired: 1 in]
                    }
                  }
                }
                n170 = property on="IMAQDevice Mode" class="Ring (strict)"(error in=w718, "Strings []"=w719) -> (error out=w717:errorcluster)  [unwired: 1 in, 1 out]
              }
              frame Enabled {
              }
            }
          }
          event "Snap": Value Change {
            n171 = event-data() -> ()  [unwired: 1 in, 5 out]
            n172 = call "BaseProcess.call process 2.vi"("i ref in"=w743, "Object"=w742, "Selector"="snap_and_publish", "error in (no error)"=w745) -> ("error out"=w744:errorcluster)  [unwired: 14 in, 1 out]
          }
          event "stop": Value Change {
            n173 = event-data() -> ()  [unwired: 1 in, 6 out]
          }
        }
        n174 = Unbundle By Name(w534) -> ("status"=w533:bool, "code"=w532:i32, "source"=w529:string)
        n175 = local write "Error"(w533) -> ()
        n176 = Number To Decimal String(number=w532) -> (decimal integer string=w530:string)  [unwired: 1 in]
        n177 = Concatenate Strings(w530, " : " ("string"), w529) -> (w528:string)
        n178 = local write "ErrorString"(w528) -> ()
        "loop counter" <- w545
      }
      n179 = disable-structure shown="Disabled" {
        disable-tunnel: w152 -> [w451 _]
        disable-tunnel: w153 -> [w450 _]
        disable-tunnel: w156 -> [w449 _]
        disable-tunnel: w158 -> [w448 _]
        disable-tunnel: w165 -> [w445 _]
        frame Disabled {
          n180 = while {
            tunnel: w451 -> [w468]
            tunnel: w450 -> [w467]
            tunnel: w449 -> [w464]
            shift-right: [w452] -> w446
            shift-left: w448 -> [w453]
            tunnel: [w461] -> w447
            shift-right: [w456] -> _
            shift-left: w445 -> [w457]
            i -> [w455]
            stop <- w459 stop-if-true
            n181 = Increment(x=w455) -> (x+1=→"2nd loop":i32)
            n182 = local read "Grab"() -> (w466:bool)
            n183 = case shown="True" w466 {
              tunnel: [w472 w482] -> w463
              tunnel: [w471 w477] -> w462
              tunnel: w467 -> [_ w481]
              tunnel: w468 -> [_ w480]
              tunnel: w453 -> [w470 w479]
              tunnel: [w469 w478] -> w452
              frame False {
                n184 = for {
                  tunnel: w470 -> [w476] mode=indexing
                  tunnel: [w475] -> w469 mode=indexing
                  shift-right: [w474] -> w471
                  shift-left: w472 -> [w473]
                  n185 = Cancel Notification(0:w476, 3:w473) -> (8:w475:refnum<notifier>, 11:w474:errorcluster)  [unwired: 1 out]
                }
              }
              frame True {
                n186 = stacked-sequence {
                  tunnel: w482 -> [_ _]
                  tunnel: w481 -> [w483 _]
                  tunnel: w480 -> [_ _]
                  tunnel: w479 -> [_ _]
                  tunnel: [_ _] -> w478
                  tunnel: [_ _] -> w477
                  frame #0 {
                  }
                  frame #1 {
                    n187 = Wait Until Next ms Multiple(millisecond multiple=u32 1000) -> ()  [unwired: 1 out]
                  }
                }
              }
            }
            n188 = local read "Compression mode?"() -> (w465:bool)
            n189 = case "Normal Mode Image Update" shown="False" w465 {
              tunnel: w462 -> [w485 w515]
              tunnel: w452 -> [w486 _]
              tunnel: [w496 w515] -> w460
              tunnel: w464 -> [w495 w514]
              tunnel: [w494 w514] -> w461
              tunnel: w457 -> [w488 w513]
              tunnel: [w487 w513] -> w456
              frame False {
                n190 = call "IMAQController.GetNormalImage.vi"("Array"=w486, "error in"=w485) -> ("Abbruch durch Asynch"=→"Abbruch durch Asynch":bool, "Abbruch?"=w491:bool, "ImageData"=w498:i16[], "Image length"=w492:i32, "Image hight"=w493:i32, "Time stamp"=w489:i16[], "error out"=w497:errorcluster)  [unwired: 9 in, 2 out]
                "Abbruch?" <- w491
                n191 = case shown="False" w491 {
                  tunnel: w498 -> [w509 _]
                  tunnel: w493 -> [w508 _]
                  tunnel: w492 -> [w507 _]
                  tunnel: w497 -> [w505 w512]
                  tunnel: [w501 w512] -> w496
                  tunnel: w495 -> [w504 w511]
                  tunnel: [w502 w511] -> w494
                  tunnel: w489 -> [w503 _]
                  tunnel: w488 -> [w500 w510]
                  tunnel: [w499 w510] -> w487
                  frame False {
                    n192 = Reshape Array(w509, w508, w507) -> (w506:i16[][])
                    n193 = Increment(x=w500) -> (x+1=w499:i32)
                    n194 = call "IMAQ ArrayToImage"("error in (no error)"=w505, "Image Pixels (U8)"=w506, "Image"=w504) -> ("error out"=w501:errorcluster, "Image Out"=w502:T4)  [unwired: 7 in]
                    "TimeStamp Data" <- w503
                  }
                  frame True {
                  }
                }
              }
              frame True {
              }
            }
            "error out 3" <- w460
            "accepted update 2nd loop" <- w456
            n195 = Wait Until Next ms Multiple(millisecond multiple=u32 3000) -> ()  [unwired: 1 out]
            n196 = local read "stop"() -> (w459:bool)
          }
        }
        frame Enabled {
        }
      }
      n197 = while {
        tunnel: w158 -> [w190]
        tunnel: [w190] -> w154
        shift-right: [w198] -> _
        shift-left: 0 -> [w199]
        tunnel: w156 -> [w195]
        tunnel: [w196] -> w155
        shift-right: [w193] -> _
        shift-left: w163 -> [w194]
        shift-right: [w192] -> _
        shift-left: w162 -> [w191]
        shift-right: [w188] -> _
        shift-left: 0 -> [w189]
        shift-right: [w186] -> _
        shift-left: 0 ("DIM service length / byte") -> [w187]
        shift-right: [w184] -> _
        shift-left: w159 -> [w185]
        shift-right: [w182] -> _
        shift-left: w159 -> [w183]
        shift-right: [w180] -> _
        shift-left: "error out 2" -> [w197]
        tunnel: w153 -> [w179]
        tunnel: w152 -> [w178]
        stop <- w181 stop-if-true
        n198 = stacked-sequence {
          seq-local: [w200 _] -> [_ w211]
          tunnel: w199 -> [_ w235]
          tunnel: [_ w234] -> w198
          tunnel: w197 -> [_ w233]
          tunnel: [_ w232] -> w196
          tunnel: w195 -> [_ w231]
          tunnel: w194 -> [_ w230]
          tunnel: [_ w229] -> w193
          tunnel: [_ w226] -> w192
          tunnel: w191 -> [_ w225]
          tunnel: w190 -> [w203 _]
          tunnel: w189 -> [_ w223]
          tunnel: [_ w222] -> w188
          tunnel: w187 -> [_ w221]
          tunnel: [_ w219] -> w186
          tunnel: w185 -> [_ w218]
          tunnel: [_ w212] -> w184
          tunnel: w183 -> [_ w217]
          tunnel: [_ w215] -> w182
          tunnel: [_ w214] -> w181
          tunnel: [_ w213] -> w180
          tunnel: w179 -> [w205 _]
          tunnel: w178 -> [w204 _]
          frame #0 {
            n199 = for {
              tunnel: w203 -> [w210] mode=indexing
              tunnel: [w209] -> w200 mode=indexing
              shift-right: [w208] -> w202
              shift-left: errorcluster {"status"=FALSE, "code"=0, "source"=""} ("error out") -> [w207]
              n200 = Flush Queue(queue=w210, error in (no error)=w207) -> (queue out=w209:refnum<queue>, error out=w208:errorcluster)  [unwired: 1 out]
            }
            n201 = call "BaseProcess.call process 2.vi"("i ref in"=w205, "Object"=w204, "Selector"="snap_and_publish", "error in (no error)"=w202) -> ()  [unwired: 14 in, 2 out]
          }
          frame #1 {
            n202 = case shown="True" w230 {
              tunnel: w211 -> [w267 w387]
              tunnel: w235 -> [w278 w397]
              tunnel: [w277 w396] -> w234
              tunnel: w233 -> [w276 w395]
              tunnel: [w275 w394] -> w213
              tunnel: w217 -> [w274 w393]
              selector: w230 -> [w273 w384]
              tunnel: [w272 w383] -> w229
              tunnel: [w271 w382] -> w228
              tunnel: [w270 w381] -> w227
              tunnel: w225 -> [_ w380]
              tunnel: [TRUE w380] -> w224
              tunnel: w223 -> [w265 w379]
              tunnel: [w264 w378] -> w222
              tunnel: w221 -> [w263 w377]
              tunnel: [w262 w376] -> w220
              tunnel: [w260 w375] -> w212
              tunnel: w218 -> [w261 w374]
              tunnel: [w259 w373] -> w216
              frame True {
                w268 = 1  # aktueller Service
                n203 = Array Size(array=w267) -> (size(s)=w266:i32)
                n204 = while {
                  tunnel: w267 -> [w291]
                  tunnel: w273 -> [w295]
                  tunnel: [w294] -> w272
                  tunnel: [w293] -> w271
                  tunnel: [w292] -> w270
                  shift-right: [w302] -> w259
                  shift-left: w274 -> [w301]
                  shift-right: [w303] -> w275
                  shift-left: w276 -> [w304]
                  shift-right: [w287] -> _
                  shift-left: w268 -> [w289]
                  tunnel: w266 -> [w286]
                  shift-right: [w305] -> w277
                  shift-left: w278 -> [w306]
                  shift-right: [w283] -> w264
                  shift-left: w265 -> [w284]
                  shift-right: [w281] -> w262
                  shift-left: w263 -> [w282]
                  tunnel: w261 -> [w280]
                  tunnel: [w279] -> w260
                  stop <- w288 stop-if-true
                  # "andere DIM service\n(werden nur nach erstem abgefragt)"
                  n205 = Index Array(array=w291, index=w289) -> (element=w290:refnum<queue>)
                  n206 = Dequeue Element(queue=w290, timeout in ms (-1)=2000, error in (no error)=w304) -> (element=w298:i8[], timed out?=w299:bool, error out=w297:errorcluster)  [unwired: 1 out]
                  n207 = case "timed out?" shown="False" w299 {
                    tunnel: [w324 w372] -> w305
                    tunnel: w306 -> [w325 w372]
                    tunnel: w298 -> [w322 _]
                    tunnel: w297 -> [w321 w371]
                    tunnel: [w320 w371] -> w303
                    tunnel: [w319 _] -> w296
                    tunnel: w295 -> [w318 w370]
                    tunnel: [w317 w370] -> w294
                    tunnel: [w316 _] -> w293
                    tunnel: [w315 _] -> w292
                    tunnel: w289 -> [w314 w369]
                    tunnel: [w313 w369] -> w287
                    tunnel: w284 -> [w312 w368]
                    tunnel: [w311 w368] -> w283
                    tunnel: w282 -> [w310 w367]
                    tunnel: [w309 w367] -> w281
                    tunnel: w280 -> [w308 w366]
                    tunnel: [w307 w366] -> w279
                    frame False {
                      n208 = call "LVDimInterface.dim_unfold_data.vi"("rawData"=w322, "error in (no error)"=w321) -> ("data"=w323:i8[], "callBackID"=w316:i32, "no link"=w315:bool, "error out"=w320:errorcluster)  [unwired: 14 in]
                      n209 = case "no link?" shown="False" w315 {
                        tunnel: w325 -> [w338 w365]
                        tunnel: [w338 w365] -> w324
                        tunnel: w323 -> [w333 _]
                        tunnel: [w343 _] -> w319
                        tunnel: w318 -> [_ w364]
                        tunnel: [w342 w364] -> w317
                        tunnel: w314 -> [w341 w363]
                        tunnel: [w340 w363] -> w313
                        tunnel: w312 -> [w339 w362]
                        tunnel: [w337 w362] -> w311
                        tunnel: w310 -> [w336 w361]
                        tunnel: [w335 w361] -> w309
                        tunnel: w308 -> [w328 w360]
                        tunnel: [w327 w360] -> w307
                        frame False {
                          n210 = Type Cast(type=i16[] [], x=w333) -> (*(type *) &x=w330:i16[])
                          n211 = Split 1D Array(array=w330, index=3) -> (first subarray=w329:i16[], second subarray=w331:i16[])
                          n212 = Equal?(x=w328, y=w329) -> ()  [unwired: 1 out]
                          n213 = case shown="True" TRUE {
                            tunnel: w331 -> [_ w351]
                            tunnel: [_ w351] -> w343
                            tunnel: [FALSE FALSE] -> w342
                            tunnel: w341 -> [w346 w358]
                            tunnel: [w346 w357] -> w340
                            tunnel: w339 -> [w348 w356]
                            tunnel: [w347 w355] -> w337
                            tunnel: w336 -> [w345 w354]
                            tunnel: [w345 w352] -> w335
                            tunnel: w328 -> [w344 w350]
                            tunnel: [w344 w350] -> w327
                            frame False {
                              n214 = Increment(x=w348) -> (x+1=w347:i32)
                            }
                            frame True {
                              n215 = Array Size(array=w351) -> (size(s)=w353:i32)
                              n216 = Add(x=w353, y=w354) -> (x+y=w352:i32)
                              n217 = Increment(x=w356) -> (x+1=w355:i32)
                              n218 = Increment(x=w358) -> (x+1=w357:i32)
                            }
                          }
                        }
                        frame True {
                        }
                      }
                    }
                    frame True {
                    }
                  }
                  n219 = Increment(x=w287) -> (x+1=w285:i32)
                  n220 = Greater?(x=w285, y=w286) -> (0:w288:bool)
                  n221 = Insert Into Array(array=w301, new element=w296) -> (w302:i16[])  [unwired: 1 in]
                  "receivedCounter 2" <- w284
                  "aktueller\nService" <- w289
                }
              }
              frame False {
                # "erster DIM service\n(auf diesen wird gewartet, bis er aktualisiert wurde)"
                n222 = Index Array(array=w387, index=0) -> (element=w385:refnum<queue>)
                n223 = Dequeue Element(queue=w385, timeout in ms (-1)=2000, error in (no error)=w395) -> (element=w390:i8[], timed out?=w391:bool, error out=w389:errorcluster)  [unwired: 1 out]
                n224 = case "timed out?" shown="False" w391 {
                  tunnel: [w413 w444] -> w396
                  tunnel: w397 -> [w414 w444]
                  tunnel: w390 -> [w411 _]
                  tunnel: w389 -> [w410 w443]
                  tunnel: [w409 w443] -> w394
                  tunnel: [w408 _] -> w388
                  tunnel: w384 -> [w407 w442]
                  tunnel: [w406 w442] -> w383
                  tunnel: [w404 _] -> w382
                  tunnel: [w405 _] -> w381
                  tunnel: w379 -> [w403 w441]
                  tunnel: [w402 w441] -> w378
                  tunnel: w377 -> [w401 w440]
                  tunnel: [w400 w440] -> w376
                  tunnel: [w399 w439] -> w375
                  tunnel: w374 -> [w398 w439]
                  frame False {
                    n225 = call "LVDimInterface.dim_unfold_data.vi"("rawData"=w411, "error in (no error)"=w410) -> ("data"=w412:i8[], "callBackID"=w404:i32, "no link"=w405:bool, "error out"=w409:errorcluster)  [unwired: 14 in]
                    n226 = case "no link?" shown="False" w405 {
                      tunnel: w414 -> [w433 w438]
                      tunnel: [w432 w438] -> w413
                      tunnel: w412 -> [w431 _]
                      tunnel: [w426 _] -> w408
                      tunnel: w407 -> [_ w437]
                      tunnel: [TRUE w437] -> w406
                      tunnel: w403 -> [w422 w436]
                      tunnel: [w422 w436] -> w402
                      tunnel: w401 -> [w421 w435]
                      tunnel: [w419 w435] -> w400
                      tunnel: [w415 w434] -> w399
                      tunnel: w398 -> [_ w434]
                      frame False {
                        n227 = Type Cast(type=i16[] [], x=w431) -> (*(type *) &x=w430:i16[])
                        n228 = Increment(x=w433) -> (x+1=w432:i32)
                        n229 = Array Size(array=w430) -> (size(s)=w420:i32)
                        n230 = Split 1D Array(array=w430, index=5) -> (first subarray=w416:i16[], second subarray=w426:i16[])
                        n231 = Add(x=w420, y=w421) -> (x+y=w419:i32)
                        n232 = Split 1D Array(array=w416, index=3) -> (first subarray=w415:i16[], second subarray=w417:i16[])
                        n233 = Index Array(array=w417, index #1=0 ("index")) -> (element #1=→"Image hight":i16, element #2=→"Image length":i16)  [unwired: 1 in]
                      }
                      frame True {
                      }
                    }
                  }
                  frame True {
                  }
                }
                n234 = Insert Into Array(array=w393, new element=w388) -> (w373:i16[])  [unwired: 1 in]
                "receivedCounter" <- w397
              }
            }
            "callBackID" <- w228
            "no link" <- w227
            n235 = case shown="True" w224 {
              selector: w224 -> [w238 _]
              tunnel: [w239 w246] -> w232
              tunnel: w231 -> [w239 w245]
              tunnel: [w238 FALSE] -> w226
              tunnel: w220 -> [w237 w243]
              tunnel: [w237 _] -> w219
              tunnel: w216 -> [w236 w242]
              tunnel: [w236 w241] -> w215
              tunnel: w212 -> [_ w240]
              frame False {
              }
              frame True {
                n236 = stacked-sequence {
                  tunnel: [w247 _] -> w246
                  tunnel: w245 -> [w253 _]
                  tunnel: w243 -> [_ w258]
                  tunnel: w242 -> [w248 _]
                  tunnel: [_ i16[] [] ("Array")] -> w241
                  tunnel: w240 -> [_ w254]
                  frame #0 {
                    n237 = local read "Image hight"() -> (w250:i32)
                    n238 = local read "Image length"() -> (w249:i32)
                    n239 = To Unsigned Byte Integer(number=w248) -> (unsigned 8bit integer=w251:u8[])
                    n240 = Reshape Array(w251, w250, w249) -> (w252:u8[][])
                    n241 = call "IMAQ ArrayToImage"("Image Pixels (U8)"=w252, "Image"=w253) -> ("Image Out"=w247:T4)  [unwired: 8 in, 1 out]
                    n242 = local write "Actual_Image"(w247) -> ()
                  }
                  frame #1 {
                    n243 = Multiply(x=2, y=w258) -> (x*y=→"DIM service length / byte":i32)
                    "act Time Stamp" <- w254
                  }
                }
              }
            }
            n244 = local read "stop"() -> (w214:bool)
            n245 = local write "error out 2"(w213) -> ()
          }
        }
        n246 = Wait Until Next ms Multiple(millisecond multiple=u32 3000) -> ()  [unwired: 1 out]
      }
    }
    frame #4 {
      n247 = disable-structure shown="Disabled" {
        disable-tunnel: w783 -> [w787 _]
        disable-tunnel: [w786 _] -> w761
        frame Disabled {
          n248 = for {
            tunnel: w787 -> [w790] mode=indexing
            shift-right: [w789] -> w786
            shift-left: _ -> [w788]
            n249 = call "LVDimInterface.dic_release_service.vi"("callBackID"=w790, "error in (no error)"=w788) -> ("error out"=w789:errorcluster)  [unwired: 17 in]
          }
        }
        frame Enabled {
        }
      }
      n250 = for {
        tunnel: w782 -> [w793] mode=indexing
        shift-right: [w791] -> w780
        shift-left: w761 -> [w792]
        n251 = call "LVDimInterface.dic_release_service.vi"("callBackID"=w793, "error in (no error)"=w792) -> ("error out"=w791:errorcluster)  [unwired: 17 in]
      }
      n252 = control-ref of="CompressionModeLink"() -> (w781:refnum<vi>)
      n253 = call "DimIndicators.dic_release_service.vi"("controlRef"=w781, "error in (no error)"=w780) -> ("error out"=w778:errorcluster)  [unwired: 17 in]
      n254 = control-ref of="ActualImageLink(Compression Mode)"() -> (w779:refnum<vi>)
      n255 = call "DimIndicators.dic_release_service.vi"("controlRef"=w779, "error in (no error)"=w778) -> ("error out"=w776:errorcluster)  [unwired: 17 in]
      n256 = call "destroy this.vi"("i ref in"=w784, "close FP first"=TRUE) -> ()  [unwired: 17 in, 1 out]
      n257 = control-ref of="HeightLink"() -> (w777:refnum<vi>)
      n258 = call "DimIndicators.dic_release_service.vi"("controlRef"=w777, "error in (no error)"=w776) -> ("error out"=w775:errorcluster)  [unwired: 17 in]
      n259 = control-ref of="WidthLink"() -> (w774:refnum<vi>)
      n260 = control-ref of="TimeStampAnalyzerLink"() -> (w767:refnum<vi>)
      n261 = call "DimIndicators.dic_release_service.vi"("controlRef"=w774, "error in (no error)"=w775) -> ("error out"=w773:errorcluster)  [unwired: 17 in]
      n262 = control-ref of="horizontalProjectionLink"() -> (w772:refnum<vi>)
      n263 = control-ref of="TimeStampAnalyzerLink"() -> (w764:refnum<vi>)
      n264 = call "DimIndicators.dic_release_service.vi"("controlRef"=w772, "error in (no error)"=w773) -> ("error out"=w771:errorcluster)  [unwired: 17 in]
      n265 = control-ref of="verticalProjectionLink"() -> (w770:refnum<vi>)
      n266 = control-ref of="NumberOfImagesLink"() -> (w763:refnum<vi>)
      n267 = call "DimIndicators.dic_release_service.vi"("controlRef"=w770, "error in (no error)"=w771) -> ("error out"=w768:errorcluster)  [unwired: 17 in]
      n268 = control-ref of="IntensityLink"() -> (w769:refnum<vi>)
      n269 = call "DimIndicators.dic_release_service.vi"("controlRef"=w769, "error in (no error)"=w768) -> ("error out"=w766:errorcluster)  [unwired: 17 in]
      n270 = call "DimIndicators.dic_release_service.vi"("controlRef"=w767, "error in (no error)"=w766) -> ("error out"=w765:errorcluster)  [unwired: 17 in]
      n271 = call "DimIndicators.dic_release_service.vi"("controlRef"=w764, "error in (no error)"=w765) -> ("error out"=w762:errorcluster)  [unwired: 17 in]
      n272 = call "DimIndicators.dic_release_service.vi"("controlRef"=w763, "error in (no error)"=w762) -> ()  [unwired: 17 in, 1 out]
    }
  }
  n273 = disable-structure "Controller Update im TimeOut" shown="Disabled" {
    disable-tunnel: [w808 _] -> _
    disable-tunnel: _ -> [w804 _]
    disable-tunnel: _ -> [w800 _]
    disable-tunnel: [w797 _] -> _
    disable-tunnel: _ -> [w796 _]
    frame Disabled {
      n274 = local read "CSSystems"() -> (w803:string[])
      n275 = call "CSSystemLib._getSystems_nw.vi"("error in (no error)"=w804) -> ("CSSystems"=w794:string[], "error out"=w799:errorcluster)  [unwired: 16 in, 1 out]
      n276 = Equal?(x=w803, y=w794) -> (x = y?=w802:bool[])
      n277 = call "CSSystemLib.ref2name.vi"("obj refnum"=w796) -> ("name"=w795:string)
      n278 = And Array Elements(Boolean array=w802) -> (logical AND=w801:bool)
      n279 = case "New CS System?" shown="False" w801 {
        tunnel: w800 -> [w817 w836]
        tunnel: w799 -> [w816 w837]
        tunnel: [w814 w837] -> w798
        tunnel: [w812 w836] -> w797
        tunnel: w794 -> [w809 _]
        tunnel: w795 -> [w810 _]
        frame False {
          n280 = for {
            tunnel: w817 -> [w835] mode=indexing
            shift-right: [w833] -> w815
            shift-left: w816 -> [w834]
            n281 = Release Notifier(notifier=w835, error in (no error)=w834) -> (error out=w833:errorcluster)  [unwired: 1 in, 2 out]
          }
          n282 = local write "CSSystems"(w809) -> ()
          n283 = for {
            shift-right: [w830] -> w814
            shift-left: w815 -> [w832]
            tunnel: i8[] [] -> [w829]
            tunnel: [w828] -> w812 mode=indexing
            tunnel: w809 -> [w823] mode=indexing
            tunnel: "_controller_" ("string") -> [w821]
            tunnel: w810 -> [w820]
            i -> [w818]
            w826 = T9 4 items=["ONCE_ONLY"=1, "TIMED"=2, "MONITORED"=4] ("serviceType")
            n284 = Number To Decimal String(number=w818) -> (decimal integer string=w819:string)  [unwired: 1 in]
            n285 = Concatenate Strings(w820, w821, w819) -> (w822:string)
            n286 = Obtain Notifier(name (unnamed)=w822, notification data type=w829, error in (no error)=w832) -> (notifier out=w828:refnum<notifier>, error out=w831:errorcluster)  [unwired: 1 in, 1 out]
            n287 = Concatenate Strings(w823, "/Instances" ("string")) -> (w825:string)
            n288 = call-poly "LVDimInterface.dic_info_service.vi"("serviceName"=w825, "notifierRef"=w828, "timeout [s]"=10, "serviceType"=w826, "error in (no error)"=w831) -> ("error out"=w830:errorcluster)  [unwired: 13 in, 1 out]
          }
        }
        frame True {
        }
      }
      n289 = call "IMAQController.SetNewController.vi"("Array"=w797, "error in"=w798) -> ("Controller Array"=w807:string[], "new list?"=w805:bool, "error out"=w806:errorcluster)  [unwired: 15 in]
      n290 = case shown="True" w805 {
        tunnel: w807 -> [_ w841]
        tunnel: w806 -> [w838 w840]
        tunnel: [w838 w839] -> w808
        frame False {
        }
        frame True {
          n291 = property on="Controller Listbox" class="LstBox (strict)"(error in=w840, "Item Names"=w841) -> (error out=w839:errorcluster)  [unwired: 1 in, 1 out]
        }
      }
    }
    frame Enabled {
    }
  }
  n292 = call "IMAQ Dispose"("Image"=w17) -> ()  [unwired: 5 in, 1 out]
  n293 = call "IMAQ Dispose"("Image"=w8) -> ()  [unwired: 5 in, 1 out]
  n294 = for {
    tunnel: w2 -> [w842] mode=indexing
    n295 = Release Notifier(notifier=w842) -> ()  [unwired: 2 in, 3 out]
  }
  n296 = for {
    tunnel: w3 -> [w843] mode=indexing
    n297 = Release Queue(queue=w843) -> ()  [unwired: 2 in, 3 out]
  }
